vi "Multiple Class_Multiple State_Original.vi"() -> ()   [LabVIEW 2021]
uses:
  Commander/Commander.lvclass
  C:/Program Files (x86)/Hyper State Machine Framework/SSW_Hyper_State_Machine.lvlibp/State_Machine_Class/Main_State_Machine/Hyper_State_Machine.lvclass
  Common_State/Common_State.lvclass
  Image_Acquisition/Image_Acquisition.lvclass
  Motion_Control/Motion_Control.lvclass
  Data_Logging/Data_Logging.lvclass
  DIO/DIO.lvclass
  C:/Program Files (x86)/Hyper State Machine Framework/SSW_Hyper_State_Machine.lvlibp/State_Machine_Class/State_Machine_Module.llb/State Machine.ctl
  C:/Program Files (x86)/Hyper State Machine Framework/SSW_Hyper_State_Machine.lvlibp/State_Machine_Class/State_Machine_Module.llb/Lock_Unlock.ctl
  C:/Program Files (x86)/Hyper State Machine Framework/SSW_Hyper_State_Machine.lvlibp/State_Machine_Class/State_Machine_Module.llb/Iterval.ctl
  C:/Program Files (x86)/Hyper State Machine Framework/SSW_Hyper_State_Machine.lvlibp/State_Machine_Class/State_Machine_Module.llb/Time_Out.ctl
  <vilib>/numeric/Random Number (Range) DBL.vi
  <vilib>/Utility/High Resolution Relative Seconds.vi
  C:/Program Files (x86)/Hyper State Machine Framework/SSW_Hyper_State_Machine.lvlibp
panel:
  out "Activate":bool
  out "Lamp":bool
  out "Current_Pos":dbl caption="mm"
  in  "EMO":bool
  out "Product ID":string
  in  "Activate_Code(Blank for 30 min Trial)":string="ROeInPkJ3DxAXwEgzbbW2XA0t1jaS1URlS9jikesQMED6VfU"
  out "Heart_Rate":bool
  out "Heart rate(s)":dbl format="%#_6p"
  out "Execute rate(Hz)":dbl format="%#_6p"
  out "Base Class_Time_Act":bool
  out "Base Class_Elapsed Time(s)":dbl format="%#_6p"
  out "Base Class":bool=TRUE
  out "Base Class_Remaining(s)":dbl format="%#_6p"
  out "Base Class Progress":dbl(slide) scale=0.0..10.0
  in  "Base Class":dbl=10.0 max=1000.0 format="%#_13p"
  out "Base Class":string
  out "Base Class_Active":bool
  in  "Action Manager":T1(ring)
  out "Common":bool=TRUE
  out "Common_State":string
  out "Common_Time_Act":bool
  out "Common_Elapsed Time(s)":dbl format="%#_6p"
  out "Common_State Progress":dbl(slide) scale=0.0..5.0
  in  "Common_State_Interval":dbl=5.0 max=1000.0 format="%#_13p"
  out "Common_State_Active":bool
  out "Common_State_Remaining(s)":dbl format="%#_6p"
  out "Data Logging Progress":dbl(slide) scale=0.0..3.0
  out "DIO Progress":dbl(slide) scale=0.0..0.01
  out "Motion Control Progress":dbl(slide) scale=0.0..0.5
  out "Image Acquisition Progress":dbl(slide) scale=0.0..0.001
  out "Commander Progress":dbl(slide)=-1.0 scale=0.0..1.0
  out "Data_Logging":bool=TRUE
  out "Data Logging":string
  out "Data_Logging_Time_Act":bool
  out "Data_Logging_Elapsed Time(s)":dbl format="%#_6p"
  out "DIO":bool=TRUE
  out "DIO":string
  out "DIO_Time_Act":bool
  out "DIO_Elapsed Time(s)":dbl format="%#_6p"
  out "Motion_Control":bool=TRUE
  out "Motion_Control":string
  out "Motion_Control_Time_Act":bool
  out "Motion_Control_Elapsed Time(s)":dbl format="%#_6p"
  in  "Data Logging":dbl=3.0 max=1000.0 format="%#_13p"
  out "Data Logging_Active":bool
  out "Data Logging_Remaining(s)":dbl format="%#_6p"
  in  "DIO_Interval":dbl=0.01 max=1000.0 format="%#_13p"
  in  "Motion_Control_Interval":dbl=0.5 max=1000.0 format="%#_13p"
  out "Motion Control_Act":bool
  out "DIO_Act":bool
  out "DIO_Remaining(s)":dbl format="%#_6p"
  out "Motion_Control_Remaining(s)":dbl format="%#_6p"
  in  "Image Acquisition_Interval":dbl=0.001 max=1000.0 format="%#_13p"
  in  "Commander_Interval":dbl max=1000.0 format="%#_13p"
  in  "System_Wait_Time":dbl=0.025 format="%#_13p"
  out "Commander_Active":bool
  out "Image Acquisition_Act":bool
  out "Image Acquisition_Remaining(s)":dbl format="%#_6p"
  out "Commander_Remaining(s)":dbl format="%#_6p"
  out "Image Acquisition":bool=TRUE
  out "Image Acquisition":string
  out "Commander":bool=TRUE
  out "Image Acquisition_Time_Act":bool
  out "Image Acquisition_Elapsed Time(s)":dbl format="%#_6p"
  out "Commander":string
  out "State1_Time_Act":bool
  out "Commander_Elapsed Time(s)":dbl format="%#_6p"
  in  "Stop":bool
  # "Note : Each State is Waiting Until Commader State Finished on \"Interval_Delay\" and then Unlock"
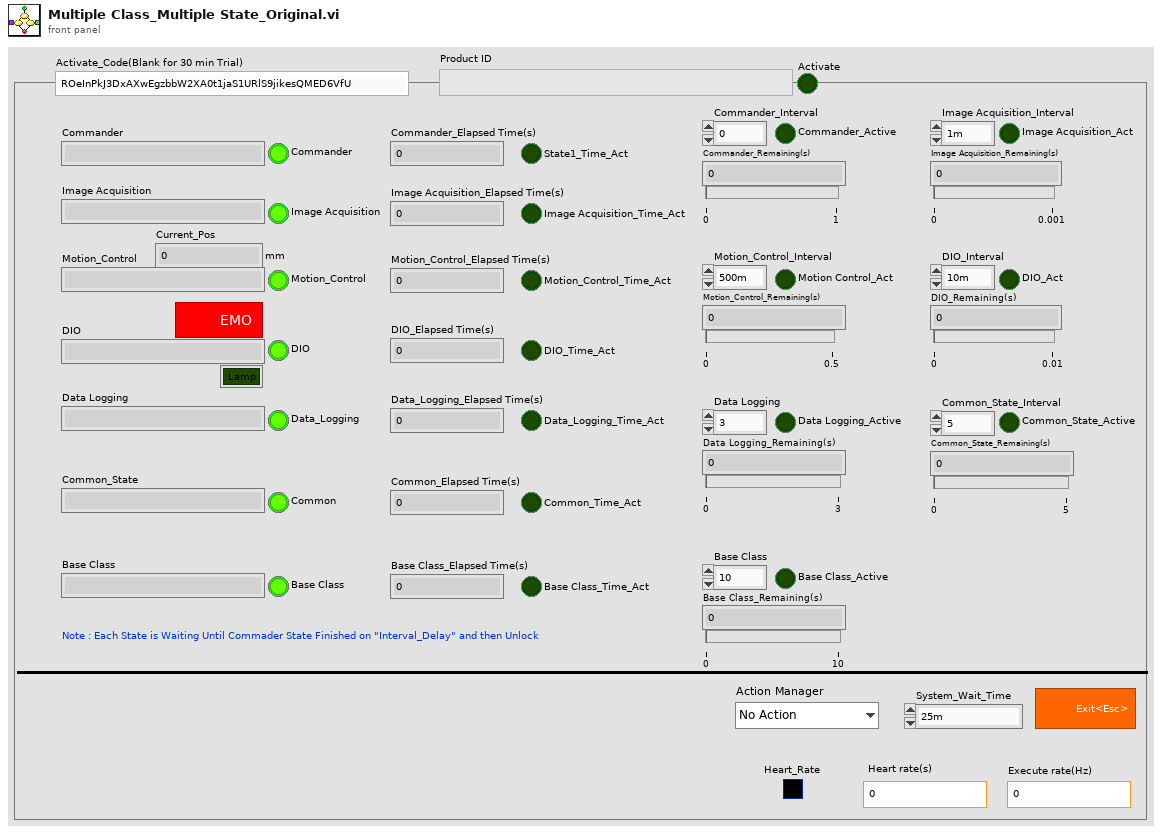
[diagram p1: front panel]
types:
  T1 = enum16{"No Action", "Init", "Lock", "Unlock", "Release"}
  T2 = typedef "SSW_Hyper_State_Machine.lvlibp/State Machine.ctl" = cluster{"Command":string, "Data":variant}
  T3 = typedef "SSW_Hyper_State_Machine.lvlibp/Time_Out.ctl" = cluster{"Enable(True)":bool, "Time Out_State Name":string, "Time Target (1s)":dbl, "Time Out_Reply Message_State":string}
  T4 = typedef "SSW_Hyper_State_Machine.lvlibp/Lock_Unlock.ctl" = cluster{"Action_Mode (Get)":enum16{"Set", "Get"}, "Action_Set (False)":bool, "State_In (Wait)":string}
  T5 = typedef "SSW_Hyper_State_Machine.lvlibp/Iterval.ctl" = cluster{"Delay(s)":dbl, "State (Interval_Delay)":string}
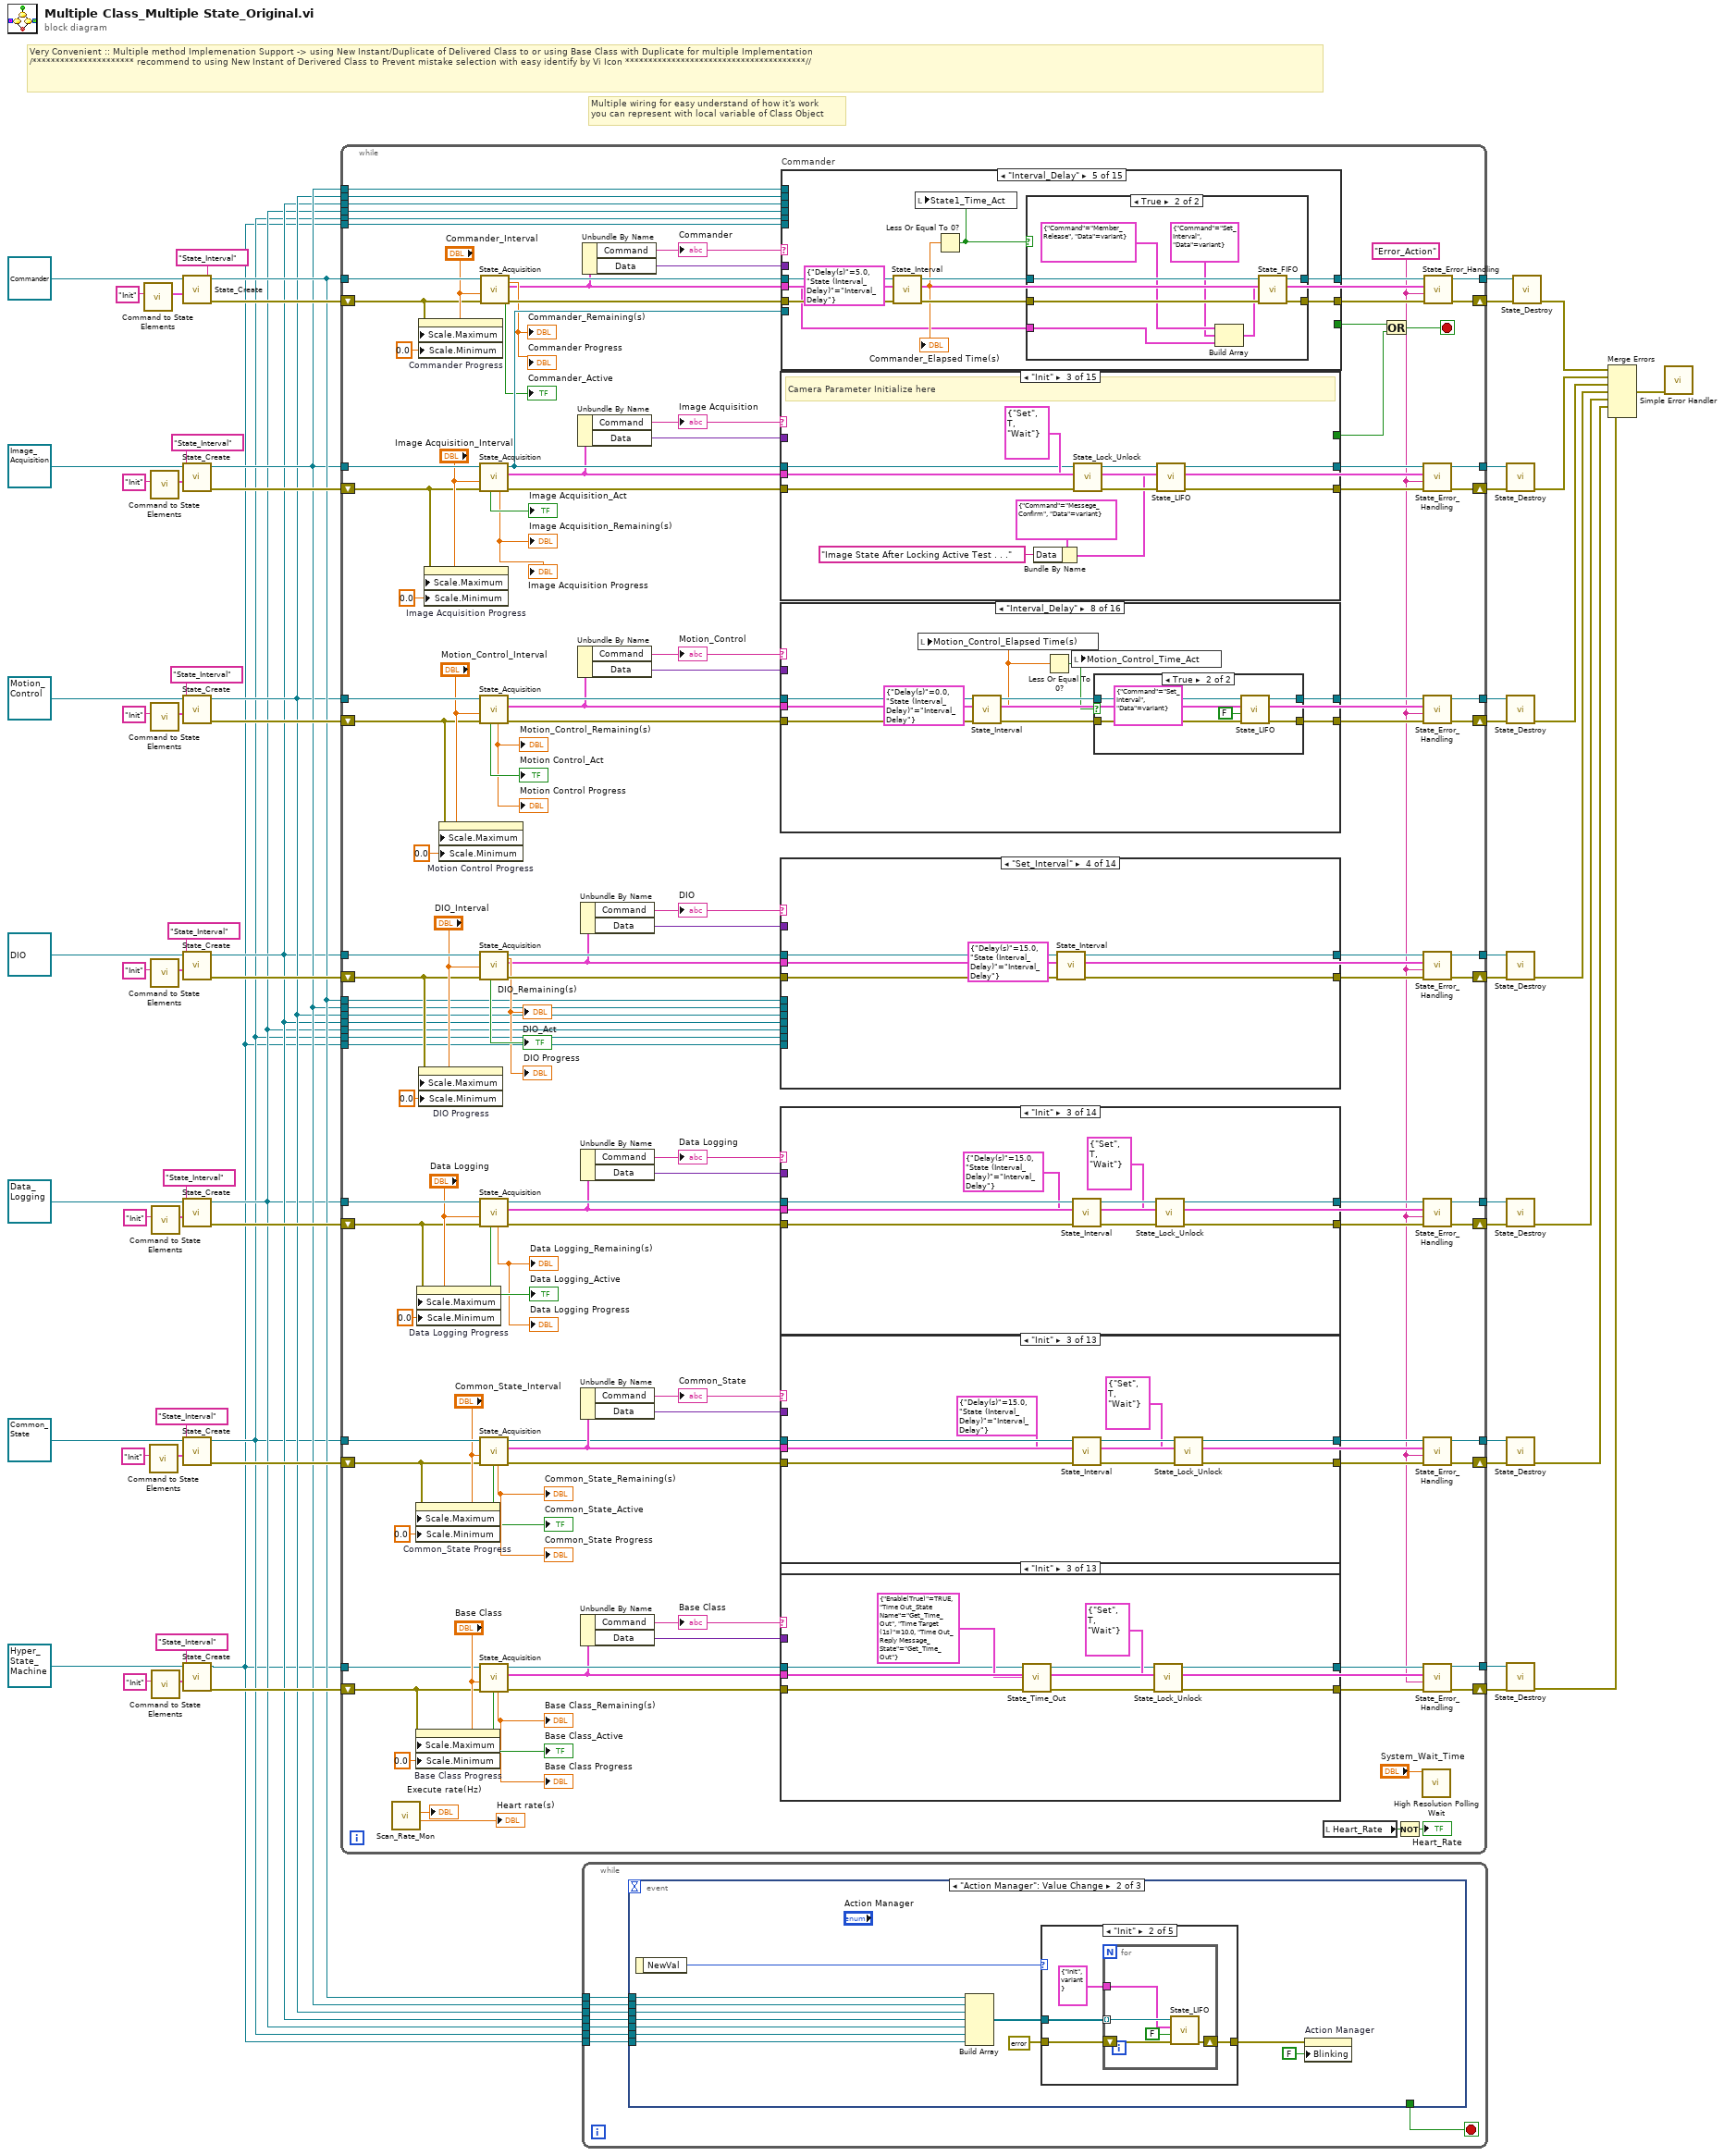
[diagram p0: block diagram]
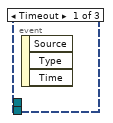
[diagram p2: hidden frame]
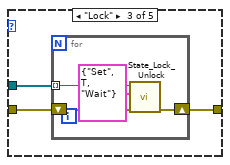
[diagram p4: hidden frame]
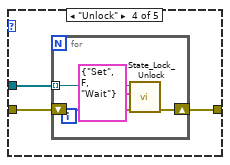
[diagram p5: hidden frame]
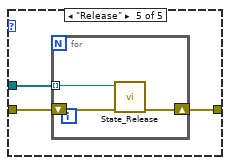
[diagram p6: hidden frame]
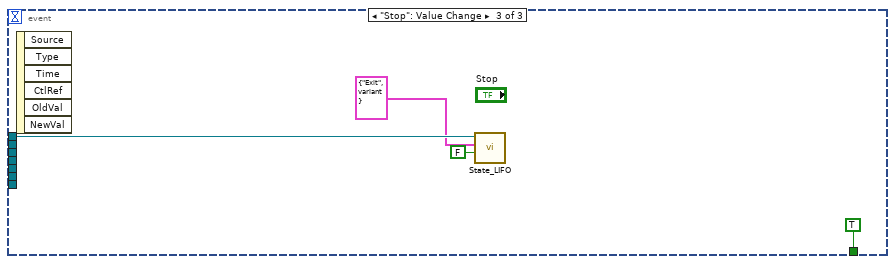
[diagram p7: hidden frame]
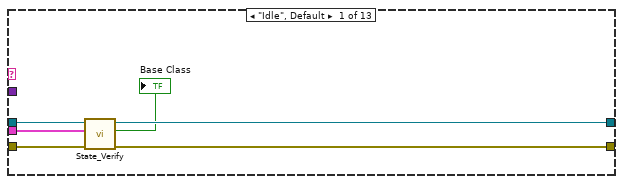
[diagram p8: hidden frame]
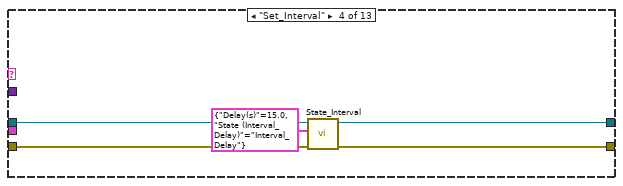
[diagram p10: hidden frame]
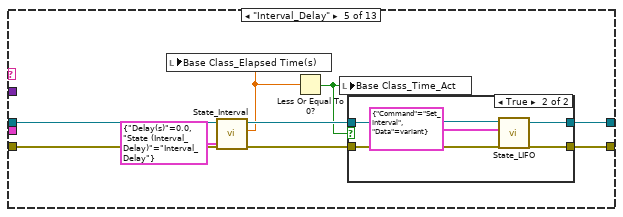
[diagram p11: hidden frame]
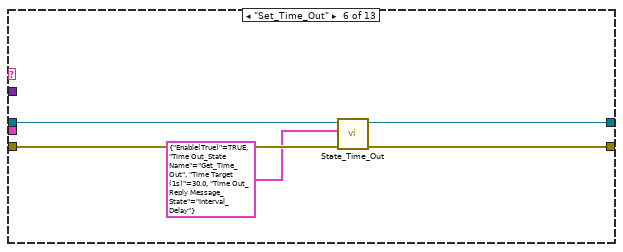
[diagram p13: hidden frame]
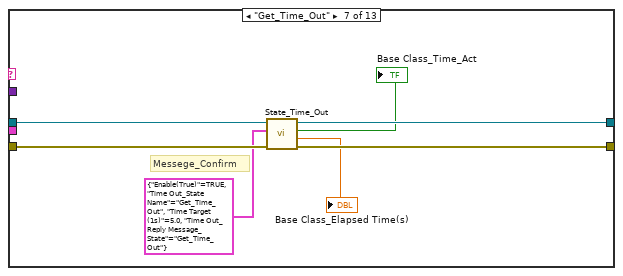
[diagram p14: hidden frame]
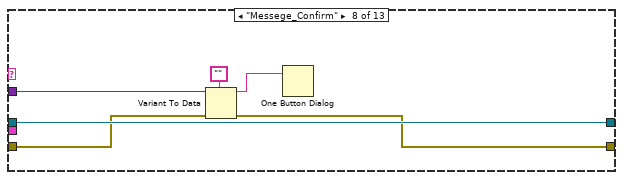
[diagram p15: hidden frame]
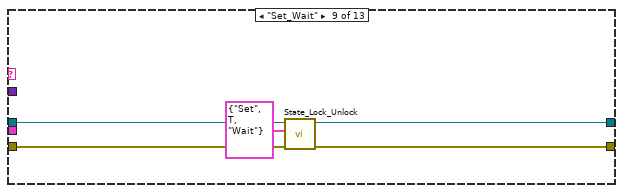
[diagram p16: hidden frame]
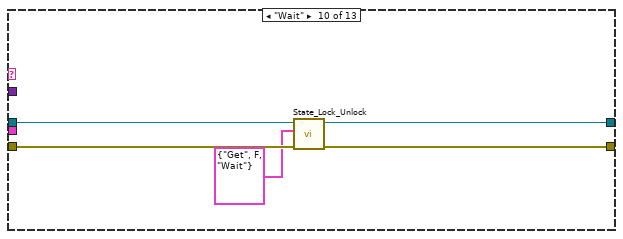
[diagram p17: hidden frame]
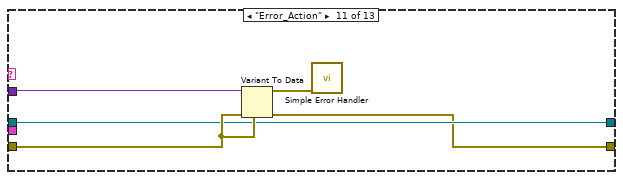
[diagram p18: hidden frame]
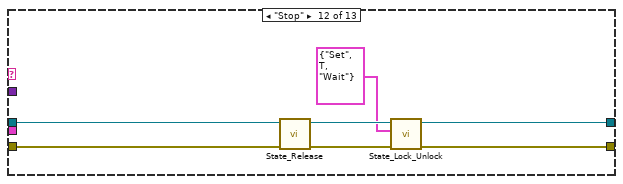
[diagram p19: hidden frame]
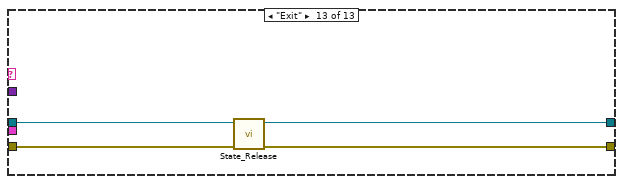
[diagram p20: hidden frame]
diagram:
  # "Multiple wiring for easy understand of how it's work\nyou can represent with local variable of Class Object"
  # "Very Convenient :: Multiple method Implemenation Support -> using New Instant/Duplicate of Delivered Class to or using Base Class with Duplicate for multiple Implementation\n/********************** recommend to using New Instant of Derivered Class to Prevent mistake selection with easy identify by Vi Icon ***************************************//"
  n1 = call "Command to State Elements.vi"("Command"="Init") -> ("Command to State Elements"=w25:T2)  [unwired: 10 in]
  n2 = call "Command to State Elements.vi"("Command"="Init") -> ("Command to State Elements"=w17:T2)  [unwired: 10 in]
  n3 = call "Command to State Elements.vi"("Command"="Init") -> ("Command to State Elements"=w27:T2)  [unwired: 10 in]
  n4 = call "Command to State Elements.vi"("Command"="Init") -> ("Command to State Elements"=w23:T2)  [unwired: 10 in]
  n5 = call "Command to State Elements.vi"("Command"="Init") -> ("Command to State Elements"=w21:T2)  [unwired: 10 in]
  n6 = call "Command to State Elements.vi"("Command"="Init") -> ("Command to State Elements"=w19:T2)  [unwired: 10 in]
  n7 = call "Command to State Elements.vi"("Command"="Init") -> ("Command to State Elements"=w15:T2)  [unwired: 10 in]
  n8 = call-dynamic "State_Create.vi"("Init_State(Option)"=w25, "State_Interval_Name"="State_Interval" ("Core_Interval_Name(State_Interval)"), "State_Machine_Class in"=refnum<class "Commander.lvclass"> refnum ("Commander.lvclass")) -> ("error out"=w64:errorcluster, "State_Machine_Class out"=w7:refnum<class "Commander.lvclass">)  [unwired: 6 in, 1 out]
  n9 = call-dynamic "State_Create.vi"("Init_State(Option)"=w27, "State_Interval_Name"="State_Interval" ("Core_Interval_Name(State_Interval)"), "State_Machine_Class in"=refnum<class "Image_Acquisition.lvclass"> refnum ("Image_Acquisition.lvclass")) -> ("error out"=w61:errorcluster, "State_Machine_Class out"=w6:refnum<class "Image_Acquisition.lvclass">)  [unwired: 6 in, 1 out]
  n10 = call-dynamic "State_Create.vi"("Init_State(Option)"=w23, "State_Interval_Name"="State_Interval" ("Core_Interval_Name(State_Interval)"), "State_Machine_Class in"=refnum<class "Motion_Control.lvclass"> refnum ("Motion_Control.lvclass")) -> ("error out"=w49:errorcluster, "State_Machine_Class out"=w5:refnum<class "Motion_Control.lvclass">)  [unwired: 6 in, 1 out]
  n11 = call-dynamic "State_Create.vi"("Init_State(Option)"=w21, "State_Interval_Name"="State_Interval" ("Core_Interval_Name(State_Interval)"), "State_Machine_Class in"=refnum<class "DIO.lvclass"> refnum ("DIO.lvclass")) -> ("error out"=w47:errorcluster, "State_Machine_Class out"=w4:refnum<class "DIO.lvclass">)  [unwired: 6 in, 1 out]
  n12 = call-dynamic "State_Create.vi"("Init_State(Option)"=w19, "State_Interval_Name"="State_Interval" ("Core_Interval_Name(State_Interval)"), "State_Machine_Class in"=refnum<class "Data_Logging.lvclass"> refnum ("Data_Logging.lvclass")) -> ("error out"=w43:errorcluster, "State_Machine_Class out"=w3:refnum<class "Data_Logging.lvclass">)  [unwired: 6 in, 1 out]
  n13 = call-dynamic "State_Create.vi"("Init_State(Option)"=w17, "State_Interval_Name"="State_Interval" ("Core_Interval_Name(State_Interval)"), "State_Machine_Class in"=refnum<class "Common_State.lvclass"> refnum ("Common_State.lvclass")) -> ("error out"=w38:errorcluster, "State_Machine_Class out"=w2:refnum<class "Common_State.lvclass">)  [unwired: 6 in, 1 out]
  n14 = call-dynamic "State_Create.vi"("Init_State(Option)"=w15, "State_Interval_Name"="State_Interval" ("Core_Interval_Name(State_Interval)"), "State_Machine_Class in"=refnum<class "Hyper_State_Machine.lvclass"> refnum ("SSW_Hyper_State_Machine.lvlibp:Hyper_State_Machine.lvclass")) -> ("error out"=w32:errorcluster, "State_Machine_Class out"=w1:refnum<class "Hyper_State_Machine.lvclass">)  [unwired: 6 in, 1 out]
  n15 = while {
    tunnel: w7 -> [w176]
    shift-right: [w185] -> w63
    shift-left: w64 -> [w84]
    tunnel: [w184] -> w62
    tunnel: w6 -> [w180]
    tunnel: [w179] -> w60
    shift-right: [w178] -> w59
    shift-left: w61 -> [w83]
    tunnel: [w154] -> w51
    tunnel: [w153] -> w50
    tunnel: w5 -> [w152]
    tunnel: w4 -> [w151]
    tunnel: w3 -> [w150]
    shift-right: [w149] -> w48
    shift-left: w49 -> [w82]
    tunnel: [w147] -> w45
    shift-right: [w148] -> w46
    shift-left: w47 -> [w81]
    shift-right: [w146] -> w44
    shift-left: w43 -> [w80]
    tunnel: w2 -> [w125]
    tunnel: [w124] -> w37
    shift-right: [w123] -> w36
    shift-left: w38 -> [w79]
    shift-right: [w93] -> w31
    shift-left: w32 -> [w78]
    tunnel: w1 -> [w97]
    tunnel: [w92] -> w30
    tunnel: w6 -> [w77]
    tunnel: w5 -> [w76]
    tunnel: w4 -> [w75]
    tunnel: w3 -> [w74]
    tunnel: w2 -> [w73]
    tunnel: w1 -> [w72]
    tunnel: w7 -> [w71]
    tunnel: w6 -> [w70]
    tunnel: w5 -> [w69]
    tunnel: w4 -> [w68]
    tunnel: w3 -> [w67]
    tunnel: w2 -> [w66]
    tunnel: w1 -> [w65]
    stop <- w175 stop-if-true
    w91 = "Error_Action" ("State_Error_Handling")
    n16 = call "Scan_Rate_Mon.vi"() -> ("Heart rate(s)"=→"Heart rate(s)":dbl, "Execute rate(Hz)"=→"Execute rate(Hz)":dbl)
    n17 = property on="Common_State Progress" class="Slide (strict)"(error in=w79, "Scale.Maximum"="Common_State_Interval", "Scale.Minimum"=0.0 ("Scale.Range:Minimum")) -> ()  [unwired: 1 in, 2 out]
    n18 = property on="Base Class Progress" class="Slide (strict)"(error in=w78, "Scale.Maximum"="Base Class", "Scale.Minimum"=0.0 ("Scale.Range:Minimum")) -> ()  [unwired: 1 in, 2 out]
    n19 = property on="Data Logging Progress" class="Slide (strict)"(error in=w80, "Scale.Maximum"="Data Logging", "Scale.Minimum"=0.0 ("Scale.Range:Minimum")) -> ()  [unwired: 1 in, 2 out]
    n20 = property on="Commander Progress" class="Slide (strict)"(error in=w84, "Scale.Maximum"="Commander_Interval", "Scale.Minimum"=0.0 ("Scale.Range:Minimum")) -> ()  [unwired: 1 in, 2 out]
    n21 = property on="DIO Progress" class="Slide (strict)"(error in=w81, "Scale.Maximum"="DIO_Interval", "Scale.Minimum"=0.0 ("Scale.Range:Minimum")) -> ()  [unwired: 1 in, 2 out]
    n22 = property on="Image Acquisition Progress" class="Slide (strict)"(error in=w83, "Scale.Maximum"="Image Acquisition_Interval", "Scale.Minimum"=0.0 ("Scale.Range:Minimum")) -> ()  [unwired: 1 in, 2 out]
    n23 = property on="Motion Control Progress" class="Slide (strict)"(error in=w82, "Scale.Maximum"="Motion_Control_Interval", "Scale.Minimum"=0.0 ("Scale.Range:Minimum")) -> ()  [unwired: 1 in, 2 out]
    n24 = call-dynamic "State_Acquisition.vi"("error in (no error)"=w83, "State_Interval_Time(s)"="Image Acquisition_Interval", "Main_Machine_State_Class in"=w180) -> ("error out"=w183:errorcluster, "State"=w110:T2, "Main_Machine_State_Class out"=w177:refnum<class "Image_Acquisition.lvclass">, "Remaining(ms)"=→"Image Acquisition_Remaining(s)" →"Image Acquisition Progress":dbl, "Current_State_Active"=→"Image Acquisition_Act":bool)  [unwired: 2 in, 2 out]
    n25 = call-dynamic "State_Acquisition.vi"("error in (no error)"=w82, "State_Interval_Time(s)"="Motion_Control_Interval", "Main_Machine_State_Class in"=w152) -> ("error out"=w156:errorcluster, "State"=w109:T2, "Main_Machine_State_Class out"=w157:refnum<class "Motion_Control.lvclass">, "Remaining(ms)"=→"Motion_Control_Remaining(s)" →"Motion Control Progress":dbl, "Current_State_Active"=→"Motion Control_Act":bool)  [unwired: 2 in, 2 out]
    n26 = call-dynamic "State_Acquisition.vi"("error in (no error)"=w81, "State_Interval_Time(s)"="DIO_Interval", "Main_Machine_State_Class in"=w151) -> ("error out"=w163:errorcluster, "State"=w108:T2, "Main_Machine_State_Class out"=w164:refnum<class "DIO.lvclass">, "Remaining(ms)"=→"DIO_Remaining(s)" →"DIO Progress":dbl, "Current_State_Active"=→"DIO_Act":bool)  [unwired: 2 in, 2 out]
    n27 = call-dynamic "State_Acquisition.vi"("error in (no error)"=w80, "State_Interval_Time(s)"="Data Logging", "Main_Machine_State_Class in"=w150) -> ("error out"=w165:errorcluster, "State"=w107:T2, "Main_Machine_State_Class out"=w166:refnum<class "Data_Logging.lvclass">, "Remaining(ms)"=→"Data Logging_Remaining(s)" →"Data Logging Progress":dbl, "Current_State_Active"=→"Data Logging_Active":bool)  [unwired: 2 in, 2 out]
    n28 = call-dynamic "State_Acquisition.vi"("error in (no error)"=w79, "State_Interval_Time(s)"="Common_State_Interval", "Main_Machine_State_Class in"=w125) -> ("error out"=w127:errorcluster, "State"=w106:T2, "Main_Machine_State_Class out"=w90:refnum<class "Common_State.lvclass">, "Remaining(ms)"=→"Common_State_Remaining(s)" →"Common_State Progress":dbl, "Current_State_Active"=→"Common_State_Active":bool)  [unwired: 2 in, 2 out]
    n29 = call-dynamic "State_Acquisition.vi"("error in (no error)"=w78, "State_Interval_Time(s)"="Base Class", "Main_Machine_State_Class in"=w97) -> ("error out"=w98:errorcluster, "State"=w95:T2, "Main_Machine_State_Class out"=w99:refnum<class "Hyper_State_Machine.lvclass">, "Remaining(ms)"=→"Base Class_Remaining(s)" →"Base Class Progress":dbl, "Current_State_Active"=→"Base Class_Active":bool)  [unwired: 2 in, 2 out]
    n30 = call-dynamic "State_Acquisition.vi"("error in (no error)"=w84, "State_Interval_Time(s)"="Commander_Interval", "Main_Machine_State_Class in"=w176) -> ("error out"=w187:errorcluster, "State"=w111:T2, "Main_Machine_State_Class out"=w188:refnum<class "Commander.lvclass">, "Remaining(ms)"=→"Commander_Remaining(s)" →"Commander Progress":dbl, "Current_State_Active"=→"Commander_Active":bool)  [unwired: 2 in, 2 out]
    n31 = Unbundle By Name(w110) -> ("Command"=w181:string, "Data"=w182:variant)
    "Image Acquisition" <- w181
    n32 = Unbundle By Name(w109) -> ("Command"=w140:string, "Data"=w169:variant)
    "Motion_Control" <- w140
    n33 = Unbundle By Name(w108) -> ("Command"=w141:string, "Data"=w168:variant)
    "DIO" <- w141
    n34 = Unbundle By Name(w107) -> ("Command"=w142:string, "Data"=w167:variant)
    "Data Logging" <- w142
    n35 = Unbundle By Name(w106) -> ("Command"=w120:string, "Data"=w126:variant)
    "Common_State" <- w120
    n36 = Unbundle By Name(w95) -> ("Command"=w103:string, "Data"=w100:variant)
    "Base Class" <- w103
    n37 = Unbundle By Name(w111) -> ("Command"=w191:string, "Data"=w190:variant)
    "Commander" <- w191
    n38 = case shown="\"Init\"" w181 {
      selector: w181 -> [_ _ _ _ w683 _ _ _ _ _ _ _ _ _ _]
      tunnel: w182 -> [_ _ _ _ _ _ _ _ _ w741 _ _ w760 _ _]
      tunnel: w177 -> [w663 w665 w674 w681 w688 w693 w706 w724 w731 w735 w751 w756 w757 w768 w773]
      tunnel: w183 -> [w662 w664 w673 w680 w687 w692 w705 w723 w730 w739 w750 w755 w759 w767 w772]
      tunnel: [w656 w665 w667 w679 w686 w691 w701 w722 w729 w736 w749 w754 w757 w763 w771] -> w171
      tunnel: [w655 w664 w666 w678 w685 w690 w700 w721 w728 w734 w748 w753 w758 w762 w770] -> w170
      tunnel: w110 -> [w661 _ _ _ _ _ _ _ _ _ _ _ _ _ _]
      tunnel: [_ _ _ _ _ _ _ _ _ _ _ _ _ _ TRUE] -> w174
      frame "Idle", Default {
        n39 = call-dynamic "State_Verify.vi"("error in (no error)"=w662, "State(Idle)"=w661, "State_Machine_Class in"=w663) -> ("error out"=w658:errorcluster, "Active"=→"Image Acquisition":bool, "State_Machine_Class out"=w659:refnum<class "Image_Acquisition.lvclass">)  [unwired: 6 in]
        n40 = Build Array(T2 {"Command"="Image_Acquisition", "Data"=variant} ("State")) -> (w654:T2[])
        n41 = call-dynamic "State_FIFO.vi"("error in (no error)"=w658, "State Machine[]"=w654, "State_Machine_Class in"=w659) -> ("error out"=w655:errorcluster, "State_Machine_Class out"=w656:refnum<class "Image_Acquisition.lvclass">)  [unwired: 7 in]
      }
      frame "State_Interval" {
      }
      frame "Init" {
        # "Camera Parameter Initialize here"
        n42 = Bundle By Name(cluster=T2 {"Command"="Messege_Confirm", "Data"=variant} ("State Machine"), "Data"="Image State After Locking Active Test . . .") -> (w669:T2)
        n43 = call-dynamic "State_Lock_Unlock.vi"("error in (no error)"=w673, "Parameter"=T4 {"Action_Mode (Get)"=enum."Set", "Action_Set (False)"=TRUE, "State_In (Wait)"="Wait"}, "State_Machine_Class in"=w674) -> ("error out"=w671:errorcluster, "State_Machine_Class out"=w672:refnum<class "Image_Acquisition.lvclass">)  [unwired: 6 in, 1 out]
        n44 = call-dynamic "State_LIFO.vi"("error in (no error)"=w671, "State Machine"=w669, "State_Machine_Class in"=w672) -> ("error out"=w666:errorcluster, "State_Machine_Class out"=w667:refnum<class "Image_Acquisition.lvclass">)  [unwired: 7 in]
      }
      frame "Test_Interval" {
        n45 = call-dynamic "State_Interval.vi"("error in (no error)"=w680, "Parameter"=T5 {"Delay(s)"=0.0, "State (Interval_Delay)"="Test_Interval"}, "State_Machine_Class in"=w681) -> ("error out"=w678:errorcluster, "Elapsed Time(s)"=w677:dbl, "State_Machine_Class out"=w679:refnum<class "Image_Acquisition.lvclass">)  [unwired: 6 in]
        n46 = local write "Image Acquisition_Elapsed Time(s)"(w677) -> ()
      }
      frame "Image_Acquisition" {
        (unwired) T5 {"Delay(s)"=5.0, "State (Interval_Delay)"="Image_Acquisition"} ("Parameter")
        # "Simple handling with specify name"
        # "Dynamic handling Name for Waiting Demo"
        # "Image Acquisition Function Here"
        n47 = Bundle By Name(cluster=T5 {"Delay(s)"=5.0, "State (Interval_Delay)"=""} ("Parameter"), "State (Interval_Delay)"=w683) -> (w682:T5)
        n48 = call-dynamic "State_Interval.vi"("error in (no error)"=w687, "Parameter"=w682, "State_Machine_Class in"=w688) -> ("error out"=w685:errorcluster, "State_Machine_Class out"=w686:refnum<class "Image_Acquisition.lvclass">)  [unwired: 6 in, 1 out]
      }
      frame "Set_Interval" {
        n49 = call-dynamic "State_Interval.vi"("error in (no error)"=w692, "Parameter"=T5 {"Delay(s)"=15.0, "State (Interval_Delay)"="Interval_Delay"}, "State_Machine_Class in"=w693) -> ("error out"=w690:errorcluster, "State_Machine_Class out"=w691:refnum<class "Image_Acquisition.lvclass">)  [unwired: 6 in, 1 out]
      }
      frame "Interval_Delay" {
        n50 = call-dynamic "State_Interval.vi"("error in (no error)"=w705, "Parameter"=T5 {"Delay(s)"=0.0, "State (Interval_Delay)"="Interval_Delay"}, "State_Machine_Class in"=w706) -> ("error out"=w702:errorcluster, "Elapsed Time(s)"=w699:dbl, "State_Machine_Class out"=w703:refnum<class "Image_Acquisition.lvclass">)  [unwired: 6 in]
        "Image Acquisition_Elapsed Time(s)" <- w699
        n51 = Build Array(T2 {"Command"="Interval_Delay", "Data"=variant} ("State"), T2 {"Command"="Image_Acquisition", "Data"=variant} ("State")) -> (w695:T2[])
        n52 = Less Or Equal To 0?(x=w699) -> (x <= 0?=w704:bool)
        n53 = Reverse 1D Array(array=w695) -> (reversed array=w694:T2[])
        n54 = case shown="True" w704 {
          tunnel: w703 -> [w708 w713]
          tunnel: w702 -> [w707 w712]
          tunnel: [w708 w711] -> w701
          tunnel: [w707 w710] -> w700
          tunnel: w694 -> [_ w709]
          frame False {
          }
          frame True {
            n55 = for {
              shift-right: [w716] -> w711
              shift-left: w713 -> [w718]
              shift-right: [w715] -> w710
              shift-left: w712 -> [w717]
              tunnel: w709 -> [w714] mode=indexing
              n56 = call-dynamic "State_LIFO.vi"("error in (no error)"=w717, "State Machine"=w714, "State_Machine_Class in"=w718) -> ("error out"=w715:errorcluster, "State_Machine_Class out"=w716:refnum<class "Image_Acquisition.lvclass">)  [unwired: 7 in]
            }
          }
        }
        n57 = local write "Image Acquisition_Time_Act"(w704) -> ()
      }
      frame "Set_Time_Out" {
        n58 = call-dynamic "State_Time_Out.vi"("error in (no error)"=w723, "Parameter"=T3 {"Enable(True)"=TRUE, "Time Out_State Name"="Get_Time_Out", "Time Target (1s)"=30.0, "Time Out_Reply Message_State"="Messege_Confirm"}, "State_Machine_Class in"=w724) -> ("error out"=w721:errorcluster, "Timeout"=w720:bool, "State_Machine_Class out"=w722:refnum<class "Image_Acquisition.lvclass">)  [unwired: 5 in, 1 out]
        n59 = local write "Image Acquisition_Time_Act"(w720) -> ()
      }
      frame "Get_Time_Out" {
        # "Messege_Confirm"
        n60 = call-dynamic "State_Time_Out.vi"("error in (no error)"=w730, "Parameter"=T3 {"Enable(True)"=TRUE, "Time Out_State Name"="Get_Time_Out", "Time Target (1s)"=0.0, "Time Out_Reply Message_State"="Messege_Confirm"}, "State_Machine_Class in"=w731) -> ("error out"=w728:errorcluster, "Remaining Time (s)"=w727:dbl, "Timeout"=→"Image Acquisition_Time_Act":bool, "State_Machine_Class out"=w729:refnum<class "Image_Acquisition.lvclass">)  [unwired: 5 in]
        n61 = local write "Image Acquisition_Elapsed Time(s)"(w727) -> ()
      }
      frame "Messege_Confirm" {
        n62 = Variant To Data(error in=w739, type="", Variant=w741) -> (data=w738:string, error out=w737:errorcluster)
        n63 = One Button Dialog(message=w738) -> (true=w732:bool)  [unwired: 1 in]
        n64 = flat-sequence {
          tunnel: w737 -> [w746]
          tunnel: [w745] -> w736
          tunnel: w735 -> [w744]
          tunnel: [w743] -> w734
          tunnel: T5 {"Delay(s)"=5.0, "State (Interval_Delay)"="Test_Interval"} ("Parameter") -> [w742]
          tunnel: w732 -> [_]
          frame #0 {
            n65 = call-dynamic "State_Interval.vi"("error in (no error)"=w746, "Parameter"=w742, "State_Machine_Class in"=w744) -> ("error out"=w743:errorcluster, "State_Machine_Class out"=w745:refnum<class "Image_Acquisition.lvclass">)  [unwired: 6 in, 1 out]
          }
        }
      }
      frame "Set_Wait" {
        n66 = call-dynamic "State_Lock_Unlock.vi"("error in (no error)"=w750, "Parameter"=T4 {"Action_Mode (Get)"=enum."Set", "Action_Set (False)"=TRUE, "State_In (Wait)"="Wait"}, "State_Machine_Class in"=w751) -> ("error out"=w748:errorcluster, "State_Machine_Class out"=w749:refnum<class "Image_Acquisition.lvclass">)  [unwired: 6 in, 1 out]
      }
      frame "Wait" {
        n67 = call-dynamic "State_Lock_Unlock.vi"("error in (no error)"=w755, "Parameter"=T4 {"Action_Mode (Get)"=enum."Get", "Action_Set (False)"=FALSE, "State_In (Wait)"="Wait"}, "State_Machine_Class in"=w756) -> ("error out"=w753:errorcluster, "State_Machine_Class out"=w754:refnum<class "Image_Acquisition.lvclass">)  [unwired: 6 in, 1 out]
      }
      frame "Error_Action" {
        n68 = Variant To Data(error in=w759, type=w759, Variant=w760) -> (data=w761:errorcluster, error out=w758:errorcluster)
        n69 = call <vilib>:"Simple Error Handler.vi"("error in (no error)"=w761) -> ()  [unwired: 4 in, 5 out]
      }
      frame "Stop" {
        n70 = call-dynamic "State_Release.vi"("error in (no error)"=w767, "State_Machine_Class in"=w768) -> ("error out"=w765:errorcluster, "State_Machine_Class out"=w766:refnum<class "Image_Acquisition.lvclass">)  [unwired: 8 in]
        n71 = call-dynamic "State_Lock_Unlock.vi"("error in (no error)"=w765, "Parameter"=T4 {"Action_Mode (Get)"=enum."Set", "Action_Set (False)"=TRUE, "State_In (Wait)"="Wait"}, "State_Machine_Class in"=w766) -> ("error out"=w762:errorcluster, "State_Machine_Class out"=w763:refnum<class "Image_Acquisition.lvclass">)  [unwired: 6 in, 1 out]
      }
      frame "Exit" {
        n72 = call-dynamic "State_Release.vi"("error in (no error)"=w772, "State_Machine_Class in"=w773) -> ("error out"=w770:errorcluster, "State_Machine_Class out"=w771:refnum<class "Image_Acquisition.lvclass">)  [unwired: 8 in]
      }
    }
    n73 = case shown="\"Interval_Delay\"" w140 {
      tunnel: w169 -> [_ _ _ _ _ _ _ _ _ _ w627 _ _ w640 _ _]
      tunnel: w157 -> [w563 w565 w571 w579 w584 w587 w592 w601 w614 w621 w625 w632 w637 w641 w649 w653]
      tunnel: w156 -> [w562 w564 w569 w578 w583 w586 w591 w600 w613 w620 w624 w631 w636 w639 w648 w652]
      tunnel: [w556 w565 w573 w577 w582 w587 w590 w597 w612 w619 w625 w630 w635 w641 w645 w651] -> w158
      tunnel: [w555 w564 w572 w576 w581 w586 w589 w596 w611 w618 w623 w629 w634 w638 w644 w650] -> w155
      tunnel: w109 -> [w561 _ _ _ _ _ _ _ _ _ _ _ _ _ _ _]
      frame "Idle", Default {
        n74 = call-dynamic "State_Verify.vi"("error in (no error)"=w562, "State(Idle)"=w561, "State_Machine_Class in"=w563) -> ("error out"=w558:errorcluster, "Active"=→"Motion_Control":bool, "State_Machine_Class out"=w559:refnum<class "Motion_Control.lvclass">)  [unwired: 6 in]
        n75 = Build Array(T2 {"Command"="Motion_Move", "Data"=variant} ("State")) -> (w554:T2[])
        n76 = call-dynamic "State_FIFO.vi"("error in (no error)"=w558, "State Machine[]"=w554, "State_Machine_Class in"=w559) -> ("error out"=w555:errorcluster, "State_Machine_Class out"=w556:refnum<class "Motion_Control.lvclass">)  [unwired: 7 in]
      }
      frame "State_Interval" {
        # "Handling Motion I/O or Cirtical Task Here"
      }
      frame "Init" {
        # "Motion Parameter Initialize Here"
        n77 = Build Array(T2 {"Command"="Motion_Move", "Data"=variant} ("State")) -> (w566:T2[])
        n78 = call-dynamic "State_FIFO.vi"("error in (no error)"=w569, "State Machine[]"=w566, "State_Machine_Class in"=w571) -> ("error out"=w568:errorcluster, "State_Machine_Class out"=w570:refnum<class "Motion_Control.lvclass">)  [unwired: 7 in]
        n79 = call-dynamic "State_Lock_Unlock.vi"("error in (no error)"=w568, "Parameter"=T4 {"Action_Mode (Get)"=enum."Set", "Action_Set (False)"=TRUE, "State_In (Wait)"="Wait"}, "State_Machine_Class in"=w570) -> ("error out"=w572:errorcluster, "State_Machine_Class out"=w573:refnum<class "Motion_Control.lvclass">)  [unwired: 6 in, 1 out]
      }
      frame "Motion_Move" {
        # "Motion Move Command here"
        n80 = call-dynamic "State_LIFO.vi"("error in (no error)"=w578, "State Machine"=T2 {"Command"="Motion_Request_Pos", "Data"=variant} ("State"), "State_Machine_Class in"=w579) -> ("error out"=w576:errorcluster, "State_Machine_Class out"=w577:refnum<class "Motion_Control.lvclass">)  [unwired: 7 in]
      }
      frame "Motion_Request_Pos" {
        # "Motion Query Position Command here"
        n81 = call-dynamic "State_LIFO.vi"("error in (no error)"=w583, "State Machine"=T2 {"Command"="Motion_Get_Pos", "Data"=variant} ("State"), "State_Machine_Class in"=w584) -> ("error out"=w581:errorcluster, "State_Machine_Class out"=w582:refnum<class "Motion_Control.lvclass">)  [unwired: 7 in]
      }
      frame "Motion_Get_Pos" {
        # "Motion Move Command here"
        n82 = call-poly <vilib>:"Random Number (Range).vi"() -> ("number"=→"Current_Pos":dbl)  [unwired: 11 in]
      }
      frame "Set_Interval" {
        n83 = call-dynamic "State_Interval.vi"("error in (no error)"=w591, "Parameter"=T5 {"Delay(s)"=15.0, "State (Interval_Delay)"="Interval_Delay"}, "State_Machine_Class in"=w592) -> ("error out"=w589:errorcluster, "State_Machine_Class out"=w590:refnum<class "Motion_Control.lvclass">)  [unwired: 6 in, 1 out]
      }
      frame "Interval_Delay" {
        n84 = call-dynamic "State_Interval.vi"("error in (no error)"=w600, "Parameter"=T5 {"Delay(s)"=0.0, "State (Interval_Delay)"="Interval_Delay"}, "State_Machine_Class in"=w601) -> ("error out"=w598:errorcluster, "Elapsed Time(s)"=w595:dbl, "State_Machine_Class out"=w599:refnum<class "Motion_Control.lvclass">)  [unwired: 6 in]
        n85 = local write "Motion_Control_Elapsed Time(s)"(w595) -> ()
        n86 = Less Or Equal To 0?(x=w595) -> (x <= 0?=w594:bool)
        n87 = local write "Motion_Control_Time_Act"(w594) -> ()
        n88 = case shown="True" w594 {
          tunnel: w599 -> [w603 w609]
          tunnel: w598 -> [w602 w608]
          tunnel: [w603 w607] -> w597
          tunnel: [w602 w606] -> w596
          frame False {
          }
          frame True {
            n89 = call-dynamic "State_LIFO.vi"("error in (no error)"=w608, "State_Interval(Enable)"=FALSE, "State Machine"=T2 {"Command"="Set_Interval", "Data"=variant} ("State"), "State_Machine_Class in"=w609) -> ("error out"=w606:errorcluster, "State_Machine_Class out"=w607:refnum<class "Motion_Control.lvclass">)  [unwired: 6 in]
          }
        }
      }
      frame "Set_Time_Out" {
        n90 = call-dynamic "State_Time_Out.vi"("error in (no error)"=w613, "Parameter"=T3 {"Enable(True)"=TRUE, "Time Out_State Name"="Get_Time_Out", "Time Target (1s)"=30.0, "Time Out_Reply Message_State"="Messege_Confirm"}, "State_Machine_Class in"=w614) -> ("error out"=w611:errorcluster, "State_Machine_Class out"=w612:refnum<class "Motion_Control.lvclass">)  [unwired: 5 in, 2 out]
      }
      frame "Get_Time_Out" {
        # "Messege_Confirm"
        n91 = call-dynamic "State_Time_Out.vi"("error in (no error)"=w620, "Parameter"=T3 {"Enable(True)"=TRUE, "Time Out_State Name"="Get_Time_Out", "Time Target (1s)"=0.0, "Time Out_Reply Message_State"="Messege_Confirm"}, "State_Machine_Class in"=w621) -> ("error out"=w618:errorcluster, "Remaining Time (s)"=→"Motion_Control_Elapsed Time(s)":dbl, "Timeout"=→"Motion_Control_Time_Act":bool, "State_Machine_Class out"=w619:refnum<class "Motion_Control.lvclass">)  [unwired: 5 in]
      }
      frame "Messege_Confirm" {
        n92 = Variant To Data(error in=w624, type="", Variant=w627) -> (data=w622:string, error out=w623:errorcluster)
        n93 = One Button Dialog(message=w622) -> ()  [unwired: 1 in, 1 out]
      }
      frame "Set_Wait" {
        n94 = call-dynamic "State_Lock_Unlock.vi"("error in (no error)"=w631, "Parameter"=T4 {"Action_Mode (Get)"=enum."Set", "Action_Set (False)"=TRUE, "State_In (Wait)"="Wait"}, "State_Machine_Class in"=w632) -> ("error out"=w629:errorcluster, "State_Machine_Class out"=w630:refnum<class "Motion_Control.lvclass">)  [unwired: 6 in, 1 out]
      }
      frame "Wait" {
        n95 = call-dynamic "State_Lock_Unlock.vi"("error in (no error)"=w636, "Parameter"=T4 {"Action_Mode (Get)"=enum."Get", "Action_Set (False)"=FALSE, "State_In (Wait)"="Wait"}, "State_Machine_Class in"=w637) -> ("error out"=w634:errorcluster, "State_Machine_Class out"=w635:refnum<class "Motion_Control.lvclass">)  [unwired: 6 in, 1 out]
      }
      frame "Error_Action" {
        n96 = Variant To Data(error in=w639, type=w639, Variant=w640) -> (data=w642:errorcluster, error out=w638:errorcluster)
        n97 = call <vilib>:"Simple Error Handler.vi"("error in (no error)"=w642) -> ()  [unwired: 4 in, 5 out]
      }
      frame "Stop" {
        n98 = call-dynamic "State_Release.vi"("error in (no error)"=w648, "State_Machine_Class in"=w649) -> ("error out"=w646:errorcluster, "State_Machine_Class out"=w647:refnum<class "Motion_Control.lvclass">)  [unwired: 8 in]
        n99 = call-dynamic "State_Lock_Unlock.vi"("error in (no error)"=w646, "Parameter"=T4 {"Action_Mode (Get)"=enum."Set", "Action_Set (False)"=TRUE, "State_In (Wait)"="Wait"}, "State_Machine_Class in"=w647) -> ("error out"=w644:errorcluster, "State_Machine_Class out"=w645:refnum<class "Motion_Control.lvclass">)  [unwired: 6 in, 1 out]
      }
      frame "Exit" {
        n100 = call-dynamic "State_Release.vi"("error in (no error)"=w652, "State_Machine_Class in"=w653) -> ("error out"=w650:errorcluster, "State_Machine_Class out"=w651:refnum<class "Motion_Control.lvclass">)  [unwired: 8 in]
      }
    }
    n101 = case shown="\"Set_Interval\"" w141 {
      tunnel: w168 -> [_ _ _ _ _ _ _ _ w524 _ _ w537 _ _]
      tunnel: w164 -> [w448 w458 w475 w490 w497 w502 w509 w515 w522 w529 w534 w535 w549 w553]
      tunnel: w163 -> [w447 w449 w474 w489 w496 w501 w508 w514 w521 w528 w533 w538 w548 w552]
      tunnel: [w442 w458 w478 w488 w492 w500 w507 w513 w522 w527 w532 w535 w545 w551] -> w162
      tunnel: [w441 w449 w477 w487 w491 w499 w506 w512 w520 w526 w531 w536 w542 w550] -> w161
      tunnel: w108 -> [w446 _ _ _ _ _ _ _ _ _ _ _ _ _]
      tunnel: w71 -> [_ w456 _ _ _ _ _ _ _ _ _ _ _ _]
      tunnel: w70 -> [_ w455 _ _ _ _ _ _ _ _ _ _ _ _]
      tunnel: w69 -> [_ w454 _ _ _ _ _ _ _ _ _ _ _ _]
      tunnel: w68 -> [_ w453 _ _ _ _ _ _ _ _ _ _ _ _]
      tunnel: w67 -> [_ w452 _ _ _ _ _ _ _ _ _ _ _ _]
      tunnel: w66 -> [_ w451 _ _ _ _ _ _ _ _ _ _ _ _]
      tunnel: w65 -> [_ w450 _ _ _ _ _ _ _ _ _ _ _ _]
      frame "Idle", Default {
        # "Able to activate at \"Stae_Interval\""
        n102 = call-dynamic "State_Verify.vi"("error in (no error)"=w447, "State(Idle)"=w446, "State_Machine_Class in"=w448) -> ("error out"=w443:errorcluster, "Active"=→"DIO":bool, "State_Machine_Class out"=w444:refnum<class "DIO.lvclass">)  [unwired: 6 in]
        n103 = Build Array(T2 {"Command"="Lamp_Blinking", "Data"=variant} ("State")) -> (w439:T2[])
        n104 = call-dynamic "State_FIFO.vi"("error in (no error)"=w443, "State Machine[]"=w439, "State_Machine_Class in"=w444) -> ("error out"=w441:errorcluster, "State_Machine_Class out"=w442:refnum<class "DIO.lvclass">)  [unwired: 7 in]
      }
      frame "State_Interval" {
        # "Able to assign to Even to handling"
        # "Simulation of Emergency Signal , Pree to try (Can not Override State Lock if in Active)"
        # "Simulation of Emergency Signal"
        # "Every Cycle Time DIO Get Data Here"
        n105 = case shown="True" "EMO" {
          tunnel: w456 -> [_ w468]
          tunnel: w455 -> [_ w467]
          tunnel: w454 -> [_ w466]
          tunnel: w453 -> [_ w465]
          tunnel: w452 -> [_ w464]
          tunnel: w451 -> [_ w463]
          tunnel: w450 -> [_ w462]
          tunnel: w449 -> [_ w459]
          frame False {
          }
          frame True {
            n106 = Build Array(w468, w467, w466, w465, w464, w463, w462) -> (w461:refnum<class "Hyper_State_Machine.lvclass">[])
            n107 = for {
              tunnel: w461 -> [w470] mode=indexing
              tunnel: T2 {"Command"="Stop", "Data"=variant} ("State") -> [w471]
              shift-right: [w473] -> _
              shift-left: w459 -> [w469]
              n108 = call-dynamic "State_LIFO.vi"("error in (no error)"=w469, "State_Interval(Enable)"=FALSE, "State Machine"=w471, "State_Machine_Class in"=w470) -> ("error out"=w473:errorcluster)  [unwired: 6 in, 1 out]
            }
          }
        }
      }
      frame "Init" {
        # "DIO Parameter Initialize here"
        n109 = disable-structure shown="Enabled" {
          disable-tunnel: [w483 w485] -> w478
          disable-tunnel: [w482 w484] -> w477
          disable-tunnel: w475 -> [w480 w485]
          disable-tunnel: w474 -> [w479 w484]
          frame Disabled {
            n110 = call-dynamic "State_Lock_Unlock.vi"("error in (no error)"=w479, "Parameter"=T4 {"Action_Mode (Get)"=enum."Set", "Action_Set (False)"=TRUE, "State_In (Wait)"="Wait"}, "State_Machine_Class in"=w480) -> ("error out"=w482:errorcluster, "State_Machine_Class out"=w483:refnum<class "DIO.lvclass">)  [unwired: 6 in, 1 out]
          }
          frame Enabled {
          }
        }
        "Lamp" <- FALSE ("Lamp")
      }
      frame "Set_Interval" {
        n111 = call-dynamic "State_Interval.vi"("error in (no error)"=w489, "Parameter"=T5 {"Delay(s)"=15.0, "State (Interval_Delay)"="Interval_Delay"}, "State_Machine_Class in"=w490) -> ("error out"=w487:errorcluster, "State_Machine_Class out"=w488:refnum<class "DIO.lvclass">)  [unwired: 6 in, 1 out]
      }
      frame "Interval_Delay" {
        n112 = call-dynamic "State_Interval.vi"("error in (no error)"=w496, "Parameter"=T5 {"Delay(s)"=0.0, "State (Interval_Delay)"="Interval_Delay"}, "State_Machine_Class in"=w497) -> ("error out"=w491:errorcluster, "Elapsed Time(s)"=w495:dbl, "State_Machine_Class out"=w492:refnum<class "DIO.lvclass">)  [unwired: 6 in]
        n113 = local write "DIO_Elapsed Time(s)"(w495) -> ()
        n114 = Less Or Equal To 0?(x=w495) -> (x <= 0?=w494:bool)
        n115 = local write "DIO_Time_Act"(w494) -> ()
      }
      frame "Set_Time_Out" {
        n116 = call-dynamic "State_Time_Out.vi"("error in (no error)"=w501, "Parameter"=T3 {"Enable(True)"=TRUE, "Time Out_State Name"="Get_Time_Out", "Time Target (1s)"=30.0, "Time Out_Reply Message_State"="Messege_Confirm"}, "State_Machine_Class in"=w502) -> ("error out"=w499:errorcluster, "State_Machine_Class out"=w500:refnum<class "DIO.lvclass">)  [unwired: 5 in, 2 out]
      }
      frame "Get_Time_Out" {
        # "Messege_Confirm"
        n117 = call-dynamic "State_Time_Out.vi"("error in (no error)"=w508, "Parameter"=T3 {"Enable(True)"=TRUE, "Time Out_State Name"="Get_Time_Out", "Time Target (1s)"=0.0, "Time Out_Reply Message_State"="Messege_Confirm"}, "State_Machine_Class in"=w509) -> ("error out"=w506:errorcluster, "Remaining Time (s)"=→"DIO_Elapsed Time(s)":dbl, "Timeout"=→"DIO_Time_Act":bool, "State_Machine_Class out"=w507:refnum<class "DIO.lvclass">)  [unwired: 5 in]
      }
      frame "Lamp_Blinking" {
        n118 = call-dynamic "State_Interval.vi"("error in (no error)"=w514, "Parameter"=T5 {"Delay(s)"=0.25, "State (Interval_Delay)"="Lamp_Blinking"}, "State_Machine_Class in"=w515) -> ("error out"=w512:errorcluster, "Elapsed Time(s)"=w510:dbl, "State_Machine_Class out"=w513:refnum<class "DIO.lvclass">)  [unwired: 6 in]
        n119 = Less Or Equal To 0?(x=w510) -> (x <= 0?=w511:bool)
        n120 = case shown="True" w511 {
          frame False {
          }
          frame True {
            n121 = local read "Lamp"() -> (w518:bool)
            n122 = Not(x=w518) -> (.not. x?=w517:bool)
            n123 = local write "Lamp"(w517) -> ()
          }
        }
      }
      frame "Messege_Confirm" {
        n124 = Variant To Data(error in=w521, type="", Variant=w524) -> (data=w519:string, error out=w520:errorcluster)
        n125 = One Button Dialog(message=w519) -> ()  [unwired: 1 in, 1 out]
      }
      frame "Set_Wait" {
        n126 = call-dynamic "State_Lock_Unlock.vi"("error in (no error)"=w528, "Parameter"=T4 {"Action_Mode (Get)"=enum."Set", "Action_Set (False)"=TRUE, "State_In (Wait)"="Wait"}, "State_Machine_Class in"=w529) -> ("error out"=w526:errorcluster, "State_Machine_Class out"=w527:refnum<class "DIO.lvclass">)  [unwired: 6 in, 1 out]
      }
      frame "Wait" {
        n127 = call-dynamic "State_Lock_Unlock.vi"("error in (no error)"=w533, "Parameter"=T4 {"Action_Mode (Get)"=enum."Get", "Action_Set (False)"=FALSE, "State_In (Wait)"="Wait"}, "State_Machine_Class in"=w534) -> ("error out"=w531:errorcluster, "State_Machine_Class out"=w532:refnum<class "DIO.lvclass">)  [unwired: 6 in, 1 out]
      }
      frame "Error_Action" {
        n128 = Variant To Data(error in=w538, type=w538, Variant=w537) -> (data=w539:errorcluster, error out=w536:errorcluster)
        n129 = call <vilib>:"Simple Error Handler.vi"("error in (no error)"=w539) -> ()  [unwired: 4 in, 5 out]
      }
      frame "Stop" {
        n130 = call-dynamic "State_Release.vi"("error in (no error)"=w548, "State_Machine_Class in"=w549) -> ("error out"=w546:errorcluster, "State_Machine_Class out"=w547:refnum<class "DIO.lvclass">)  [unwired: 8 in]
        n131 = call-dynamic "State_Lock_Unlock.vi"("error in (no error)"=w546, "Parameter"=T4 {"Action_Mode (Get)"=enum."Set", "Action_Set (False)"=TRUE, "State_In (Wait)"="Wait"}, "State_Machine_Class in"=w547) -> ("error out"=w543:errorcluster, "State_Machine_Class out"=w545:refnum<class "DIO.lvclass">)  [unwired: 6 in, 1 out]
        n132 = property on="Action Manager" class="Enum (strict)"(error in=w543, "Blinking"=TRUE) -> (error out=w542:errorcluster)  [unwired: 1 in, 1 out]
        n133 = One Button Dialog(message="All State is Locking !\nPlease Unlock With Action Manager to Release . . .") -> ()  [unwired: 1 in, 1 out]
      }
      frame "Exit" {
        n134 = call-dynamic "State_Release.vi"("error in (no error)"=w552, "State_Machine_Class in"=w553) -> ("error out"=w550:errorcluster, "State_Machine_Class out"=w551:refnum<class "DIO.lvclass">)  [unwired: 8 in]
      }
    }
    n135 = case shown="\"Init\"" w142 {
      tunnel: w167 -> [_ _ _ _ _ _ _ _ w412 _ _ w425 _ _]
      tunnel: w166 -> [w360 w362 w370 w372 w377 w386 w399 w406 w410 w417 w422 w424 w434 w438]
      tunnel: w165 -> [w359 w361 w369 w371 w376 w385 w398 w405 w409 w416 w421 w426 w433 w437]
      tunnel: [w357 w362 w366 w372 w375 w382 w397 w404 w410 w415 w420 w424 w429 w436] -> w160
      tunnel: [w356 w361 w365 w371 w374 w381 w396 w403 w408 w414 w419 w423 w428 w435] -> w159
      tunnel: w107 -> [w358 _ _ _ _ _ _ _ _ _ _ _ _ _]
      frame "Idle", Default {
        n136 = call-dynamic "State_Verify.vi"("error in (no error)"=w359, "State(Idle)"=w358, "State_Machine_Class in"=w360) -> ("error out"=w356:errorcluster, "Active"=→"Data_Logging":bool, "State_Machine_Class out"=w357:refnum<class "Data_Logging.lvclass">)  [unwired: 6 in]
      }
      frame "State_Interval" {
        # "Files Monitering or Cirtical Task Handling Here"
      }
      frame "Init" {
        n137 = call-dynamic "State_Interval.vi"("error in (no error)"=w369, "Parameter"=T5 {"Delay(s)"=15.0, "State (Interval_Delay)"="Interval_Delay"}, "State_Machine_Class in"=w370) -> ("error out"=w364:errorcluster, "State_Machine_Class out"=w367:refnum<class "Data_Logging.lvclass">)  [unwired: 6 in, 1 out]
        n138 = call-dynamic "State_Lock_Unlock.vi"("error in (no error)"=w364, "Parameter"=T4 {"Action_Mode (Get)"=enum."Set", "Action_Set (False)"=TRUE, "State_In (Wait)"="Wait"}, "State_Machine_Class in"=w367) -> ("error out"=w365:errorcluster, "State_Machine_Class out"=w366:refnum<class "Data_Logging.lvclass">)  [unwired: 6 in, 1 out]
      }
      frame "Data_Logging" {
        # "Save Data Files Here"
      }
      frame "Set_Interval" {
        n139 = call-dynamic "State_Interval.vi"("error in (no error)"=w376, "Parameter"=T5 {"Delay(s)"=15.0, "State (Interval_Delay)"="Interval_Delay"}, "State_Machine_Class in"=w377) -> ("error out"=w374:errorcluster, "State_Machine_Class out"=w375:refnum<class "Data_Logging.lvclass">)  [unwired: 6 in, 1 out]
      }
      frame "Interval_Delay" {
        n140 = call-dynamic "State_Interval.vi"("error in (no error)"=w385, "Parameter"=T5 {"Delay(s)"=0.0, "State (Interval_Delay)"="Interval_Delay"}, "State_Machine_Class in"=w386) -> ("error out"=w383:errorcluster, "Elapsed Time(s)"=w380:dbl, "State_Machine_Class out"=w384:refnum<class "Data_Logging.lvclass">)  [unwired: 6 in]
        n141 = local write "Data_Logging_Elapsed Time(s)"(w380) -> ()
        n142 = Less Or Equal To 0?(x=w380) -> (x <= 0?=w379:bool)
        n143 = local write "Data_Logging_Time_Act"(w379) -> ()
        n144 = case shown="True" w379 {
          tunnel: w384 -> [w388 w394]
          tunnel: w383 -> [w387 w393]
          tunnel: [w388 w392] -> w382
          tunnel: [w387 w391] -> w381
          frame False {
          }
          frame True {
            n145 = call-dynamic "State_LIFO.vi"("error in (no error)"=w393, "State_Interval(Enable)"=FALSE, "State Machine"=T2 {"Command"="Set_Interval", "Data"=variant} ("State"), "State_Machine_Class in"=w394) -> ("error out"=w391:errorcluster, "State_Machine_Class out"=w392:refnum<class "Data_Logging.lvclass">)  [unwired: 6 in]
          }
        }
      }
      frame "Set_Time_Out" {
        n146 = call-dynamic "State_Time_Out.vi"("error in (no error)"=w398, "Parameter"=T3 {"Enable(True)"=TRUE, "Time Out_State Name"="Get_Time_Out", "Time Target (1s)"=30.0, "Time Out_Reply Message_State"="Interval_Delay"}, "State_Machine_Class in"=w399) -> ("error out"=w396:errorcluster, "State_Machine_Class out"=w397:refnum<class "Data_Logging.lvclass">)  [unwired: 5 in, 2 out]
      }
      frame "Get_Time_Out" {
        # "Messege_Confirm"
        n147 = call-dynamic "State_Time_Out.vi"("error in (no error)"=w405, "Parameter"=T3 {"Enable(True)"=TRUE, "Time Out_State Name"="Get_Time_Out", "Time Target (1s)"=0.0, "Time Out_Reply Message_State"="Messege_Confirm"}, "State_Machine_Class in"=w406) -> ("error out"=w403:errorcluster, "Remaining Time (s)"=→"Data_Logging_Elapsed Time(s)":dbl, "Timeout"=→"Data_Logging_Time_Act":bool, "State_Machine_Class out"=w404:refnum<class "Data_Logging.lvclass">)  [unwired: 5 in]
      }
      frame "Messege_Confirm" {
        n148 = Variant To Data(error in=w409, type="", Variant=w412) -> (data=w407:string, error out=w408:errorcluster)
        n149 = One Button Dialog(message=w407) -> ()  [unwired: 1 in, 1 out]
      }
      frame "Set_Wait" {
        n150 = call-dynamic "State_Lock_Unlock.vi"("error in (no error)"=w416, "Parameter"=T4 {"Action_Mode (Get)"=enum."Set", "Action_Set (False)"=TRUE, "State_In (Wait)"="Wait"}, "State_Machine_Class in"=w417) -> ("error out"=w414:errorcluster, "State_Machine_Class out"=w415:refnum<class "Data_Logging.lvclass">)  [unwired: 6 in, 1 out]
      }
      frame "Wait" {
        n151 = call-dynamic "State_Lock_Unlock.vi"("error in (no error)"=w421, "Parameter"=T4 {"Action_Mode (Get)"=enum."Get", "Action_Set (False)"=TRUE, "State_In (Wait)"="Wait"}, "State_Machine_Class in"=w422) -> ("error out"=w419:errorcluster, "State_Machine_Class out"=w420:refnum<class "Data_Logging.lvclass">)  [unwired: 6 in, 1 out]
      }
      frame "Error_Action" {
        n152 = Variant To Data(error in=w426, type=w426, Variant=w425) -> (data=w427:errorcluster, error out=w423:errorcluster)
        n153 = call <vilib>:"Simple Error Handler.vi"("error in (no error)"=w427) -> ()  [unwired: 4 in, 5 out]
      }
      frame "Stop" {
        n154 = call-dynamic "State_Release.vi"("error in (no error)"=w433, "State_Machine_Class in"=w434) -> ("error out"=w431:errorcluster, "State_Machine_Class out"=w432:refnum<class "Data_Logging.lvclass">)  [unwired: 8 in]
        n155 = call-dynamic "State_Lock_Unlock.vi"("error in (no error)"=w431, "Parameter"=T4 {"Action_Mode (Get)"=enum."Set", "Action_Set (False)"=TRUE, "State_In (Wait)"="Wait"}, "State_Machine_Class in"=w432) -> ("error out"=w428:errorcluster, "State_Machine_Class out"=w429:refnum<class "Data_Logging.lvclass">)  [unwired: 6 in, 1 out]
      }
      frame "Exit" {
        n156 = call-dynamic "State_Release.vi"("error in (no error)"=w437, "State_Machine_Class in"=w438) -> ("error out"=w435:errorcluster, "State_Machine_Class out"=w436:refnum<class "Data_Logging.lvclass">)  [unwired: 8 in]
      }
    }
    n157 = case shown="\"Init\"" w120 {
      tunnel: w126 -> [_ _ _ _ _ _ _ w328 _ _ w342 _ _]
      tunnel: w90 -> [w278 w280 w288 w293 w294 w315 w322 w326 w333 w338 w340 w350 w354]
      tunnel: w127 -> [w277 w279 w287 w292 w302 w314 w321 w325 w332 w337 w341 w349 w353]
      tunnel: [w275 w280 w282 w291 w299 w313 w320 w326 w331 w336 w340 w345 w352] -> w128
      tunnel: [w274 w279 w281 w290 w298 w312 w319 w324 w330 w335 w339 w344 w351] -> w129
      tunnel: w106 -> [w276 _ _ _ _ _ _ _ _ _ _ _ _]
      frame "Idle", Default {
        n158 = call-dynamic "State_Verify.vi"("error in (no error)"=w277, "State(Idle)"=w276, "State_Machine_Class in"=w278) -> ("error out"=w274:errorcluster, "Active"=→"Common":bool, "State_Machine_Class out"=w275:refnum<class "Common_State.lvclass">)  [unwired: 6 in]
      }
      frame "State_Interval" {
        # "Cirtical Task Handling Here"
      }
      frame "Init" {
        n159 = call-dynamic "State_Interval.vi"("error in (no error)"=w287, "Parameter"=T5 {"Delay(s)"=15.0, "State (Interval_Delay)"="Interval_Delay"}, "State_Machine_Class in"=w288) -> ("error out"=w284:errorcluster, "State_Machine_Class out"=w285:refnum<class "Common_State.lvclass">)  [unwired: 6 in, 1 out]
        n160 = call-dynamic "State_Lock_Unlock.vi"("error in (no error)"=w284, "Parameter"=T4 {"Action_Mode (Get)"=enum."Set", "Action_Set (False)"=TRUE, "State_In (Wait)"="Wait"}, "State_Machine_Class in"=w285) -> ("error out"=w281:errorcluster, "State_Machine_Class out"=w282:refnum<class "Common_State.lvclass">)  [unwired: 6 in, 1 out]
      }
      frame "Set_Interval" {
        n161 = call-dynamic "State_Interval.vi"("error in (no error)"=w292, "Parameter"=T5 {"Delay(s)"=15.0, "State (Interval_Delay)"="Interval_Delay"}, "State_Machine_Class in"=w293) -> ("error out"=w290:errorcluster, "State_Machine_Class out"=w291:refnum<class "Common_State.lvclass">)  [unwired: 6 in, 1 out]
      }
      frame "Interval_Delay" {
        n162 = call-dynamic "State_Interval.vi"("error in (no error)"=w302, "Parameter"=T5 {"Delay(s)"=5.0, "State (Interval_Delay)"="Interval_Delay"}, "State_Machine_Class in"=w294) -> ("error out"=w300:errorcluster, "Elapsed Time(s)"=w297:dbl, "State_Machine_Class out"=w301:refnum<class "Common_State.lvclass">)  [unwired: 6 in]
        n163 = local write "Common_Elapsed Time(s)"(w297) -> ()
        n164 = Less Or Equal To 0?(x=w297) -> (x <= 0?=w296:bool)
        n165 = local write "Common_Time_Act"(w296) -> ()
        n166 = case shown="True" w296 {
          tunnel: w301 -> [w304 w310]
          tunnel: w300 -> [w303 w309]
          tunnel: [w304 w308] -> w299
          tunnel: [w303 w307] -> w298
          frame False {
          }
          frame True {
            n167 = call-dynamic "State_LIFO.vi"("error in (no error)"=w309, "State_Interval(Enable)"=FALSE, "State Machine"=T2 {"Command"="Interval_Delay", "Data"=variant} ("State"), "State_Machine_Class in"=w310) -> ("error out"=w307:errorcluster, "State_Machine_Class out"=w308:refnum<class "Common_State.lvclass">)  [unwired: 6 in]
          }
        }
      }
      frame "Set_Time_Out" {
        n168 = call-dynamic "State_Time_Out.vi"("error in (no error)"=w314, "Parameter"=T3 {"Enable(True)"=TRUE, "Time Out_State Name"="Get_Time_Out", "Time Target (1s)"=30.0, "Time Out_Reply Message_State"="Interval_Delay"}, "State_Machine_Class in"=w315) -> ("error out"=w312:errorcluster, "State_Machine_Class out"=w313:refnum<class "Common_State.lvclass">)  [unwired: 5 in, 2 out]
      }
      frame "Get_Time_Out" {
        # "Messege_Confirm"
        # "Messege_Confirm"
        n169 = call-dynamic "State_Time_Out.vi"("error in (no error)"=w321, "Parameter"=T3 {"Enable(True)"=TRUE, "Time Out_State Name"="Get_Time_Out", "Time Target (1s)"=0.0, "Time Out_Reply Message_State"="Set_Interval"}, "State_Machine_Class in"=w322) -> ("error out"=w319:errorcluster, "Remaining Time (s)"=→"Common_Elapsed Time(s)":dbl, "Timeout"=→"Common_Time_Act":bool, "State_Machine_Class out"=w320:refnum<class "Common_State.lvclass">)  [unwired: 5 in]
      }
      frame "Messege_Confirm" {
        n170 = Variant To Data(error in=w325, type="", Variant=w328) -> (data=w323:string, error out=w324:errorcluster)
        n171 = One Button Dialog(message=w323) -> ()  [unwired: 1 in, 1 out]
      }
      frame "Set_Wait" {
        n172 = call-dynamic "State_Lock_Unlock.vi"("error in (no error)"=w332, "Parameter"=T4 {"Action_Mode (Get)"=enum."Set", "Action_Set (False)"=TRUE, "State_In (Wait)"="Wait"}, "State_Machine_Class in"=w333) -> ("error out"=w330:errorcluster, "State_Machine_Class out"=w331:refnum<class "Common_State.lvclass">)  [unwired: 6 in, 1 out]
      }
      frame "Wait" {
        n173 = call-dynamic "State_Lock_Unlock.vi"("error in (no error)"=w337, "Parameter"=T4 {"Action_Mode (Get)"=enum."Get", "Action_Set (False)"=FALSE, "State_In (Wait)"="Wait"}, "State_Machine_Class in"=w338) -> ("error out"=w335:errorcluster, "State_Machine_Class out"=w336:refnum<class "Common_State.lvclass">)  [unwired: 6 in, 1 out]
      }
      frame "Error_Action" {
        n174 = Variant To Data(error in=w341, type=w341, Variant=w342) -> (data=w343:errorcluster, error out=w339:errorcluster)
        n175 = call <vilib>:"Simple Error Handler.vi"("error in (no error)"=w343) -> ()  [unwired: 4 in, 5 out]
      }
      frame "Stop" {
        n176 = call-dynamic "State_Release.vi"("error in (no error)"=w349, "State_Machine_Class in"=w350) -> ("error out"=w347:errorcluster, "State_Machine_Class out"=w348:refnum<class "Common_State.lvclass">)  [unwired: 8 in]
        n177 = call-dynamic "State_Lock_Unlock.vi"("error in (no error)"=w347, "Parameter"=T4 {"Action_Mode (Get)"=enum."Set", "Action_Set (False)"=TRUE, "State_In (Wait)"="Wait"}, "State_Machine_Class in"=w348) -> ("error out"=w344:errorcluster, "State_Machine_Class out"=w345:refnum<class "Common_State.lvclass">)  [unwired: 6 in, 1 out]
      }
      frame "Exit" {
        n178 = call-dynamic "State_Release.vi"("error in (no error)"=w353, "State_Machine_Class in"=w354) -> ("error out"=w351:errorcluster, "State_Machine_Class out"=w352:refnum<class "Common_State.lvclass">)  [unwired: 8 in]
      }
    }
    n179 = case shown="\"Init\"" w103 {
      tunnel: w100 -> [_ _ _ _ _ _ _ w246 _ _ w260 _ _]
      tunnel: w99 -> [w197 w199 w203 w212 w221 w233 w240 w244 w251 w256 w258 w268 w272]
      tunnel: w98 -> [w196 w198 w201 w211 w220 w232 w239 w243 w250 w255 w259 w267 w271]
      tunnel: [w194 w199 w207 w210 w217 w231 w238 w244 w249 w254 w258 w263 w270] -> w96
      tunnel: [w193 w198 w206 w209 w216 w230 w237 w242 w248 w253 w257 w262 w269] -> w94
      tunnel: w95 -> [w195 _ _ _ _ _ _ _ _ _ _ _ _]
      frame "Idle", Default {
        n180 = call-dynamic "State_Verify.vi"("error in (no error)"=w196, "State(Idle)"=w195, "State_Machine_Class in"=w197) -> ("error out"=w193:errorcluster, "Active"=→"Base Class":bool, "State_Machine_Class out"=w194:refnum<class "Hyper_State_Machine.lvclass">)  [unwired: 6 in]
      }
      frame "State_Interval" {
        # "Cirtical Task Handling Here"
      }
      frame "Init" {
        n181 = call-dynamic "State_Time_Out.vi"("error in (no error)"=w201, "Parameter"=T3 {"Enable(True)"=TRUE, "Time Out_State Name"="Get_Time_Out", "Time Target (1s)"=10.0, "Time Out_Reply Message_State"="Get_Time_Out"}, "State_Machine_Class in"=w203) -> ("error out"=w200:errorcluster, "State_Machine_Class out"=w202:refnum<class "Hyper_State_Machine.lvclass">)  [unwired: 5 in, 2 out]
        n182 = call-dynamic "State_Lock_Unlock.vi"("error in (no error)"=w200, "Parameter"=T4 {"Action_Mode (Get)"=enum."Set", "Action_Set (False)"=TRUE, "State_In (Wait)"="Wait"}, "State_Machine_Class in"=w202) -> ("error out"=w206:errorcluster, "State_Machine_Class out"=w207:refnum<class "Hyper_State_Machine.lvclass">)  [unwired: 6 in, 1 out]
      }
      frame "Set_Interval" {
        n183 = call-dynamic "State_Interval.vi"("error in (no error)"=w211, "Parameter"=T5 {"Delay(s)"=15.0, "State (Interval_Delay)"="Interval_Delay"}, "State_Machine_Class in"=w212) -> ("error out"=w209:errorcluster, "State_Machine_Class out"=w210:refnum<class "Hyper_State_Machine.lvclass">)  [unwired: 6 in, 1 out]
      }
      frame "Interval_Delay" {
        n184 = call-dynamic "State_Interval.vi"("error in (no error)"=w220, "Parameter"=T5 {"Delay(s)"=0.0, "State (Interval_Delay)"="Interval_Delay"}, "State_Machine_Class in"=w221) -> ("error out"=w218:errorcluster, "Elapsed Time(s)"=w215:dbl, "State_Machine_Class out"=w219:refnum<class "Hyper_State_Machine.lvclass">)  [unwired: 6 in]
        n185 = local write "Base Class_Elapsed Time(s)"(w215) -> ()
        n186 = Less Or Equal To 0?(x=w215) -> (x <= 0?=w214:bool)
        n187 = local write "Base Class_Time_Act"(w214) -> ()
        n188 = case shown="True" w214 {
          tunnel: w219 -> [w223 w228]
          tunnel: w218 -> [w222 w227]
          tunnel: [w223 w226] -> w217
          tunnel: [w222 w225] -> w216
          frame False {
          }
          frame True {
            n189 = call-dynamic "State_LIFO.vi"("error in (no error)"=w227, "State Machine"=T2 {"Command"="Set_Interval", "Data"=variant} ("State"), "State_Machine_Class in"=w228) -> ("error out"=w225:errorcluster, "State_Machine_Class out"=w226:refnum<class "Hyper_State_Machine.lvclass">)  [unwired: 7 in]
          }
        }
      }
      frame "Set_Time_Out" {
        n190 = call-dynamic "State_Time_Out.vi"("error in (no error)"=w232, "Parameter"=T3 {"Enable(True)"=TRUE, "Time Out_State Name"="Get_Time_Out", "Time Target (1s)"=30.0, "Time Out_Reply Message_State"="Interval_Delay"}, "State_Machine_Class in"=w233) -> ("error out"=w230:errorcluster, "State_Machine_Class out"=w231:refnum<class "Hyper_State_Machine.lvclass">)  [unwired: 5 in, 2 out]
      }
      frame "Get_Time_Out" {
        # "Messege_Confirm"
        n191 = call-dynamic "State_Time_Out.vi"("error in (no error)"=w239, "Parameter"=T3 {"Enable(True)"=TRUE, "Time Out_State Name"="Get_Time_Out", "Time Target (1s)"=5.0, "Time Out_Reply Message_State"="Get_Time_Out"}, "State_Machine_Class in"=w240) -> ("error out"=w237:errorcluster, "Remaining Time (s)"=→"Base Class_Elapsed Time(s)":dbl, "Timeout"=→"Base Class_Time_Act":bool, "State_Machine_Class out"=w238:refnum<class "Hyper_State_Machine.lvclass">)  [unwired: 5 in]
      }
      frame "Messege_Confirm" {
        n192 = Variant To Data(error in=w243, type="", Variant=w246) -> (data=w241:string, error out=w242:errorcluster)
        n193 = One Button Dialog(message=w241) -> ()  [unwired: 1 in, 1 out]
      }
      frame "Set_Wait" {
        n194 = call-dynamic "State_Lock_Unlock.vi"("error in (no error)"=w250, "Parameter"=T4 {"Action_Mode (Get)"=enum."Set", "Action_Set (False)"=TRUE, "State_In (Wait)"="Wait"}, "State_Machine_Class in"=w251) -> ("error out"=w248:errorcluster, "State_Machine_Class out"=w249:refnum<class "Hyper_State_Machine.lvclass">)  [unwired: 6 in, 1 out]
      }
      frame "Wait" {
        n195 = call-dynamic "State_Lock_Unlock.vi"("error in (no error)"=w255, "Parameter"=T4 {"Action_Mode (Get)"=enum."Get", "Action_Set (False)"=FALSE, "State_In (Wait)"="Wait"}, "State_Machine_Class in"=w256) -> ("error out"=w253:errorcluster, "State_Machine_Class out"=w254:refnum<class "Hyper_State_Machine.lvclass">)  [unwired: 6 in, 1 out]
      }
      frame "Error_Action" {
        n196 = Variant To Data(error in=w259, type=w259, Variant=w260) -> (data=w261:errorcluster, error out=w257:errorcluster)
        n197 = call <vilib>:"Simple Error Handler.vi"("error in (no error)"=w261) -> ()  [unwired: 4 in, 5 out]
      }
      frame "Stop" {
        n198 = call-dynamic "State_Release.vi"("error in (no error)"=w267, "State_Machine_Class in"=w268) -> ("error out"=w265:errorcluster, "State_Machine_Class out"=w266:refnum<class "Hyper_State_Machine.lvclass">)  [unwired: 8 in]
        n199 = call-dynamic "State_Lock_Unlock.vi"("error in (no error)"=w265, "Parameter"=T4 {"Action_Mode (Get)"=enum."Set", "Action_Set (False)"=TRUE, "State_In (Wait)"="Wait"}, "State_Machine_Class in"=w266) -> ("error out"=w262:errorcluster, "State_Machine_Class out"=w263:refnum<class "Hyper_State_Machine.lvclass">)  [unwired: 6 in, 1 out]
      }
      frame "Exit" {
        n200 = call-dynamic "State_Release.vi"("error in (no error)"=w271, "State_Machine_Class in"=w272) -> ("error out"=w269:errorcluster, "State_Machine_Class out"=w270:refnum<class "Hyper_State_Machine.lvclass">)  [unwired: 8 in]
      }
    }
    n201 = case "Commander" shown="\"Interval_Delay\"" w191 {
      tunnel: w190 -> [_ _ _ _ _ _ _ w844 w852 _ _ _ w878 _ _]
      tunnel: w188 -> [w779 w781 w788 w806 w816 w831 w838 w842 w848 w862 w870 w874 w879 w886 w891]
      tunnel: w187 -> [w777 w780 w787 w805 w815 w830 w837 w841 w851 _ w869 w873 w875 w885 w890]
      tunnel: [w776 w781 w790 w804 w811 w829 w836 w842 w848 w862 w868 w872 w879 w882 w889] -> w112
      tunnel: [w775 w780 w789 w803 w810 w828 w835 w840 w847 w861 w867 w871 w876 w881 w888] -> w186
      tunnel: [_ _ _ _ _ _ _ _ _ _ _ _ _ _ TRUE] -> w189
      tunnel: w111 -> [w778 _ _ _ w807 _ _ _ _ _ _ _ _ _ _]
      tunnel: w177 -> [_ _ _ _ _ _ _ _ _ _ _ _ _ _ _]
      tunnel: w77 -> [_ _ _ _ _ _ _ _ _ w859 _ _ _ _ _]
      tunnel: w76 -> [_ _ _ _ _ _ _ _ _ w858 _ _ _ _ _]
      tunnel: w75 -> [_ _ _ _ _ _ _ _ _ w857 _ _ _ _ _]
      tunnel: w74 -> [_ _ _ _ _ _ _ _ _ w856 _ _ _ _ _]
      tunnel: w73 -> [_ _ _ _ _ _ _ _ _ w855 _ _ _ _ _]
      tunnel: w72 -> [_ _ _ _ _ _ _ _ _ w854 _ _ _ _ _]
      frame "Idle", Default {
        n202 = call-dynamic "State_Verify.vi"("error in (no error)"=w777, "State(Idle)"=w778, "State_Machine_Class in"=w779) -> ("error out"=w775:errorcluster, "Active"=→"Commander":bool, "State_Machine_Class out"=w776:refnum<class "Commander.lvclass">)  [unwired: 6 in]
      }
      frame "State_Interval" {
      }
      frame "Init" {
        # "Test Using Static Delay (2s) + SetInterval (3s) = 5 sec"
        n203 = call-dynamic "Product_Activate.vi"("error in (no error)"=w787, "Activate Code"="Activate_Code(Blank for 30 min Trial)", "Commander in"=w788) -> ("error out"=w785:errorcluster, "Activate"=→"Activate":bool, "Product ID"=→"Product ID":string, "Commander out"=w786:refnum<class "Commander.lvclass">)  [unwired: 5 in]
        n204 = disable-structure shown="Enabled" {
          disable-tunnel: [w795 w800] -> w790
          disable-tunnel: [w794 w799] -> w789
          disable-tunnel: w786 -> [w792 w801]
          disable-tunnel: w785 -> [w791 w798]
          frame Disabled {
            n205 = call-dynamic "State_Interval.vi"("error in (no error)"=w791, "Parameter"=T5 {"Delay(s)"=5.0, "State (Interval_Delay)"="Interval_Delay"}, "State_Machine_Class in"=w792) -> ("error out"=w794:errorcluster, "State_Machine_Class out"=w795:refnum<class "Commander.lvclass">)  [unwired: 6 in, 1 out]
          }
          frame Enabled {
            n206 = Build Array(T2 {"Command"="Interval_Delay", "Data"=variant} ("State")) -> (w796:T2[])
            n207 = call-dynamic "State_FIFO.vi"("error in (no error)"=w798, "State Machine[]"=w796, "State_Machine_Class in"=w801) -> ("error out"=w799:errorcluster, "State_Machine_Class out"=w800:refnum<class "Commander.lvclass">)  [unwired: 7 in]
          }
        }
      }
      frame "Set_Interval" {
        n208 = call-dynamic "State_Interval.vi"("error in (no error)"=w805, "Parameter"=T5 {"Delay(s)"=3.0, "State (Interval_Delay)"="Interval_Delay"}, "State_Machine_Class in"=w806) -> ("error out"=w803:errorcluster, "State_Machine_Class out"=w804:refnum<class "Commander.lvclass">)  [unwired: 6 in, 1 out]
      }
      frame "Interval_Delay" {
        n209 = call-dynamic "State_Interval.vi"("error in (no error)"=w815, "Parameter"=T5 {"Delay(s)"=5.0, "State (Interval_Delay)"="Interval_Delay"}, "State_Machine_Class in"=w816) -> ("error out"=w812:errorcluster, "Elapsed Time(s)"=w809:dbl, "State_Machine_Class out"=w813:refnum<class "Commander.lvclass">)  [unwired: 6 in]
        "Commander_Elapsed Time(s)" <- w809
        n210 = Less Or Equal To 0?(x=w809) -> (x <= 0?=w814:bool)
        n211 = local write "State1_Time_Act"(w814) -> ()
        n212 = case shown="True" w814 {
          tunnel: w813 -> [w818 w826]
          tunnel: w812 -> [w817 w825]
          tunnel: [w818 w824] -> w811
          tunnel: [w817 w823] -> w810
          tunnel: w807 -> [_ w819]
          frame False {
          }
          frame True {
            n213 = Build Array(T2 {"Command"="Member_Release", "Data"=variant} ("State"), T2 {"Command"="Set_Interval", "Data"=variant} ("State"), w819) -> (w822:T2[])
            n214 = call-dynamic "State_FIFO.vi"("error in (no error)"=w825, "State Machine[]"=w822, "State_Machine_Class in"=w826) -> ("error out"=w823:errorcluster, "State_Machine_Class out"=w824:refnum<class "Commander.lvclass">)  [unwired: 7 in]
          }
        }
      }
      frame "Set_Time_Out" {
        n215 = call-dynamic "State_Time_Out.vi"("error in (no error)"=w830, "Parameter"=T3 {"Enable(True)"=TRUE, "Time Out_State Name"="Get_Time_Out", "Time Target (1s)"=30.0, "Time Out_Reply Message_State"="Messege_Confirm"}, "State_Machine_Class in"=w831) -> ("error out"=w828:errorcluster, "State_Machine_Class out"=w829:refnum<class "Commander.lvclass">)  [unwired: 5 in, 2 out]
      }
      frame "Get_Time_Out" {
        n216 = call-dynamic "State_Time_Out.vi"("error in (no error)"=w837, "Parameter"=T3 {"Enable(True)"=TRUE, "Time Out_State Name"="Get_Time_Out", "Time Target (1s)"=0.0, "Time Out_Reply Message_State"="Messege_Confirm"}, "State_Machine_Class in"=w838) -> ("error out"=w835:errorcluster, "Remaining Time (s)"=w834:dbl, "Timeout"=→"State1_Time_Act":bool, "State_Machine_Class out"=w836:refnum<class "Commander.lvclass">)  [unwired: 5 in]
        n217 = local write "Commander_Elapsed Time(s)"(w834) -> ()
      }
      frame "Messege_Confirm" {
        n218 = Variant To Data(error in=w841, type="", Variant=w844) -> (data=w839:string, error out=w840:errorcluster)
        n219 = One Button Dialog(message=w839) -> ()  [unwired: 1 in, 1 out]
      }
      frame "Dynamics_Release" {
        n220 = Variant To Data(error in=w851, type=refnum<class "Hyper_State_Machine.lvclass"> refnum ("SSW_Hyper_State_Machine.lvlibp:Hyper_State_Machine.lvclass"), Variant=w852) -> (data=w850:refnum<class "Hyper_State_Machine.lvclass">, error out=w849:errorcluster)
        n221 = call-dynamic "State_Lock_Unlock.vi"("error in (no error)"=w849, "Parameter"=T4 {"Action_Mode (Get)"=enum."Set", "Action_Set (False)"=FALSE, "State_In (Wait)"="Wait"}, "State_Machine_Class in"=w850) -> ("error out"=w847:errorcluster)  [unwired: 6 in, 2 out]
      }
      frame "Member_Release" {
        n222 = Build Array(w859, w858, w857, w856, w855, w854) -> (w853:refnum<class "Hyper_State_Machine.lvclass">[])
        n223 = for {
          tunnel: [w865] -> w861
          tunnel: T4 {"Action_Mode (Get)"=enum."Set", "Action_Set (False)"=FALSE, "State_In (Wait)"="Wait"} ("Parameter") -> [w864]
          tunnel: w853 -> [w863] mode=indexing
          n224 = call-dynamic "State_Lock_Unlock.vi"("Parameter"=w864, "State_Machine_Class in"=w863) -> ("error out"=w865:errorcluster)  [unwired: 7 in, 2 out]
        }
      }
      frame "Set_Wait" {
        n225 = call-dynamic "State_Lock_Unlock.vi"("error in (no error)"=w869, "Parameter"=T4 {"Action_Mode (Get)"=enum."Set", "Action_Set (False)"=TRUE, "State_In (Wait)"="Wait"}, "State_Machine_Class in"=w870) -> ("error out"=w867:errorcluster, "State_Machine_Class out"=w868:refnum<class "Commander.lvclass">)  [unwired: 6 in, 1 out]
      }
      frame "Wait" {
        n226 = call-dynamic "State_Lock_Unlock.vi"("error in (no error)"=w873, "State_Machine_Class in"=w874) -> ("error out"=w871:errorcluster, "State_Machine_Class out"=w872:refnum<class "Commander.lvclass">)  [unwired: 7 in, 1 out]
      }
      frame "Error_Action" {
        n227 = Variant To Data(error in=w875, type=w875, Variant=w878) -> (data=w877:errorcluster, error out=w876:errorcluster)
        n228 = call <vilib>:"Simple Error Handler.vi"("error in (no error)"=w877) -> ()  [unwired: 4 in, 5 out]
      }
      frame "Stop" {
        n229 = call-dynamic "State_Release.vi"("error in (no error)"=w885, "State_Machine_Class in"=w886) -> ("error out"=w883:errorcluster, "State_Machine_Class out"=w884:refnum<class "Commander.lvclass">)  [unwired: 8 in]
        n230 = call-dynamic "State_Lock_Unlock.vi"("error in (no error)"=w883, "Parameter"=T4 {"Action_Mode (Get)"=enum."Set", "Action_Set (False)"=TRUE, "State_In (Wait)"="Wait"}, "State_Machine_Class in"=w884) -> ("error out"=w881:errorcluster, "State_Machine_Class out"=w882:refnum<class "Commander.lvclass">)  [unwired: 6 in, 1 out]
      }
      frame "Exit" {
        n231 = call-dynamic "State_Release.vi"("error in (no error)"=w890, "State_Machine_Class in"=w891) -> ("error out"=w888:errorcluster, "State_Machine_Class out"=w889:refnum<class "Commander.lvclass">)  [unwired: 8 in]
      }
    }
    n232 = local read "Heart_Rate"() -> (w88:bool)
    n233 = Or(x=w189, y=w174) -> (x .or. y?=w175:bool)
    n234 = Not(x=w88) -> (.not. x?=→"Heart_Rate":bool)
    n235 = call <vilib>:"High Resolution Polling Wait.vi"("seconds to wait"="System_Wait_Time") -> ()  [unwired: 10 in, 1 out]
    n236 = call-dynamic "State_Error_Handling.vi"("error in (no error)"=w170, "Reply_State_Name"=w91, "Handling_State(State_Acquisition)"=w110, "State_Machine_Class in"=w171) -> ("error out"=w178:errorcluster, "State_Machine_Class out"=w179:refnum<class "Image_Acquisition.lvclass">)  [unwired: 6 in]
    n237 = call-dynamic "State_Error_Handling.vi"("error in (no error)"=w155, "Reply_State_Name"=w91, "Handling_State(State_Acquisition)"=w109, "State_Machine_Class in"=w158) -> ("error out"=w149:errorcluster, "State_Machine_Class out"=w154:refnum<class "Motion_Control.lvclass">)  [unwired: 6 in]
    n238 = call-dynamic "State_Error_Handling.vi"("error in (no error)"=w161, "Reply_State_Name"=w91, "Handling_State(State_Acquisition)"=w108, "State_Machine_Class in"=w162) -> ("error out"=w148:errorcluster, "State_Machine_Class out"=w153:refnum<class "DIO.lvclass">)  [unwired: 6 in]
    n239 = call-dynamic "State_Error_Handling.vi"("error in (no error)"=w159, "Reply_State_Name"=w91, "Handling_State(State_Acquisition)"=w107, "State_Machine_Class in"=w160) -> ("error out"=w146:errorcluster, "State_Machine_Class out"=w147:refnum<class "Data_Logging.lvclass">)  [unwired: 6 in]
    n240 = call-dynamic "State_Error_Handling.vi"("error in (no error)"=w129, "Reply_State_Name"=w91, "Handling_State(State_Acquisition)"=w106, "State_Machine_Class in"=w128) -> ("error out"=w123:errorcluster, "State_Machine_Class out"=w124:refnum<class "Common_State.lvclass">)  [unwired: 6 in]
    n241 = call-dynamic "State_Error_Handling.vi"("error in (no error)"=w94, "Reply_State_Name"=w91, "Handling_State(State_Acquisition)"=w95, "State_Machine_Class in"=w96) -> ("error out"=w93:errorcluster, "State_Machine_Class out"=w92:refnum<class "Hyper_State_Machine.lvclass">)  [unwired: 6 in]
    n242 = call-dynamic "State_Error_Handling.vi"("error in (no error)"=w186, "Reply_State_Name"=w91, "Handling_State(State_Acquisition)"=w111, "State_Machine_Class in"=w112) -> ("error out"=w185:errorcluster, "State_Machine_Class out"=w184:refnum<class "Commander.lvclass">)  [unwired: 6 in]
  }
  n243 = while {
    tunnel: w7 -> [w899]
    tunnel: w6 -> [w898]
    tunnel: w5 -> [w897]
    tunnel: w4 -> [w896]
    tunnel: w3 -> [w895]
    tunnel: w2 -> [w894]
    tunnel: w1 -> [w892]
    stop <- w893 stop-if-true
    n244 = event shown="[1] \"Action Manager\": Value Change" {
      selector: _ -> [_ _ _]
      dyn-events: _ -> [_ _ _]
      timeout: _ -> [_ _ _]
      tunnel: w899 -> [_ w910 w944]
      tunnel: w898 -> [_ w909 _]
      tunnel: w897 -> [_ w908 _]
      tunnel: w896 -> [_ w907 _]
      tunnel: w895 -> [_ w906 _]
      tunnel: w894 -> [_ w905 _]
      tunnel: [_ _ TRUE] -> w893
      tunnel: w892 -> [_ w903 _]
      event Timeout {
        n245 = event-data() -> ()  [unwired: 1 in, 3 out]
      }
      event "Action Manager": Value Change {
        n246 = event-data() -> ("NewVal"=w904:T1)  [unwired: 1 in]
        n247 = Build Array(w910, w909, w908, w907, w906, w905, w903) -> (w911:refnum<class "Hyper_State_Machine.lvclass">[])
        n248 = case shown="\"Init\"" w904 {
          tunnel: w911 -> [_ w916 w924 w931 w938]
          tunnel: [w912 w914 w923 w930 w936] -> w902
          tunnel: errorcluster {"status"=FALSE, "code"=0, "source"=""} ("error out") -> [w912 w915 w922 w929 w937]
          frame "No Action", Default {
          }
          frame "Init" {
            n249 = for {
              tunnel: w916 -> [w921] mode=indexing
              shift-right: [w918] -> w914
              shift-left: w915 -> [w920]
              tunnel: T2 {"Command"="Init", "Data"=variant} ("State") -> [w917]
              n250 = call-dynamic "State_LIFO.vi"("error in (no error)"=w920, "State_Interval(Enable)"=FALSE, "State Machine"=w917, "State_Machine_Class in"=w921) -> ("error out"=w918:errorcluster)  [unwired: 6 in, 1 out]
            }
          }
          frame "Lock" {
            n251 = for {
              tunnel: w924 -> [w928] mode=indexing
              shift-right: [w926] -> w923
              shift-left: w922 -> [w925]
              n252 = call-dynamic "State_Lock_Unlock.vi"("error in (no error)"=w925, "Parameter"=T4 {"Action_Mode (Get)"=enum."Set", "Action_Set (False)"=TRUE, "State_In (Wait)"="Wait"}, "State_Machine_Class in"=w928) -> ("error out"=w926:errorcluster)  [unwired: 6 in, 2 out]
            }
          }
          frame "Unlock" {
            n253 = for {
              tunnel: w931 -> [w935] mode=indexing
              shift-right: [w933] -> w930
              shift-left: w929 -> [w932]
              n254 = call-dynamic "State_Lock_Unlock.vi"("error in (no error)"=w932, "Parameter"=T4 {"Action_Mode (Get)"=enum."Set", "Action_Set (False)"=FALSE, "State_In (Wait)"="Wait"}, "State_Machine_Class in"=w935) -> ("error out"=w933:errorcluster)  [unwired: 6 in, 2 out]
            }
          }
          frame "Release" {
            n255 = for {
              tunnel: w938 -> [w941] mode=indexing
              shift-right: [w939] -> w936
              shift-left: w937 -> [w940]
              n256 = call-dynamic "State_Release.vi"("error in (no error)"=w940, "State_Machine_Class in"=w941) -> ("error out"=w939:errorcluster)  [unwired: 8 in, 1 out]
            }
          }
        }
        n257 = property on="Action Manager" class="Enum (strict)"(error in=w902, "Blinking"=FALSE) -> ()  [unwired: 1 in, 2 out]
      }
      event "Stop": Value Change {
        n258 = event-data() -> ()  [unwired: 1 in, 6 out]
        n259 = call-dynamic "State_LIFO.vi"("State_Interval(Enable)"=FALSE, "State Machine"=T2 {"Command"="Exit", "Data"=variant} ("State"), "State_Machine_Class in"=w944) -> ()  [unwired: 7 in, 2 out]
      }
    }
  }
  n260 = call-dynamic "State_Destroy.vi"("error in (no error)"=w59, "State_Machine_Class in"=w60) -> ("error out"=w57:errorcluster)  [unwired: 9 in]
  n261 = call-dynamic "State_Destroy.vi"("error in (no error)"=w48, "State_Machine_Class in"=w51) -> ("error out"=w42:errorcluster)  [unwired: 9 in]
  n262 = call-dynamic "State_Destroy.vi"("error in (no error)"=w46, "State_Machine_Class in"=w50) -> ("error out"=w41:errorcluster)  [unwired: 9 in]
  n263 = call-dynamic "State_Destroy.vi"("error in (no error)"=w44, "State_Machine_Class in"=w45) -> ("error out"=w40:errorcluster)  [unwired: 9 in]
  n264 = call-dynamic "State_Destroy.vi"("error in (no error)"=w36, "State_Machine_Class in"=w37) -> ("error out"=w35:errorcluster)  [unwired: 9 in]
  n265 = call-dynamic "State_Destroy.vi"("error in (no error)"=w31, "State_Machine_Class in"=w30) -> ("error out"=w29:errorcluster)  [unwired: 9 in]
  n266 = call-dynamic "State_Destroy.vi"("error in (no error)"=w63, "State_Machine_Class in"=w62) -> ("error out"=w58:errorcluster)  [unwired: 9 in]
  n267 = Merge Errors(w58, w57, w42, w41, w40, w35, w29) -> (w56:errorcluster)
  n268 = call <vilib>:"Simple Error Handler.vi"("error in (no error)"=w56) -> ()  [unwired: 4 in, 5 out]
